vi "Configure Experiment.vi"(8 "Error In":errorcluster, 9 "KH":T4 {"KH #" items=["A 1", "A 2", "A 3", "A 4", "A 5", "A 6", "A 7", "A 8"]}, 10 "Lockin":T6 {"Label" items=["", "I+", "I-", "V1+", "V1-", "V2+", "V2-", "V3+", "V3-", "V4+", "V4-", "dV1", "dV2", "dV3", "Vsg", "Vbg", "Vtg"]}) -> (0 "Error Out":errorcluster)   [LabVIEW 2019, in "Control Experiment.lvclass"]
doc: "Use this VI to help configure your experiment.\n1. Configure the Electrode control to show which electrode is connected to which lockin channel;\n2. Choose a Label for each electrode to configure Krohn Hite amplifier automatically\n3. Easily set all Krohn Hite channels to be \"all ground\" or \"all differential\" mode\n4. Fill out information about you and your device in the lower left corner\n5. When you are finished, or when you want to update the amplifiers, click the \"CREATE OUTPUT\" button located in upper right. Clicking this button will set the amplifiers, and write information to a functional global variable that you can easily read from elsewhere in your program"
uses:
  Control Experiment.lvclass
  Typedefs/KH Mode-enum.ctl
  Typedefs/Control Experiment JSON--cluster.ctl
  <userlib>/LevyLab/Configuration/Configuration.lvclass
  Typedefs/UI Controls --cluster.ctl
  Typedefs/Instrument Types--enum.ctl
  Typedefs/Instruments--cluster.ctl
  <userlib>/LevyLab/Krohn Hite 7008/KH7008/typedefs/shunt--enum.ctl
  <userlib>/LevyLab/Krohn Hite 7008/KH7008/KH7008.lvlib
  <userlib>/LevyLab/Krohn Hite 7008/KH7008/typedefs/gain--enum.ctl
  <userlib>/LevyLab/Krohn Hite 7008/KH7008/typedefs/Input--Enum.ctl
  <userlib>/LevyLab/Krohn Hite 7008/KH7008/typedefs/channel--numeric.ctl
  <userlib>/LevyLab/Krohn Hite 7008/KH7008/typedefs/couple--Enum.ctl
  <userlib>/LevyLab/Krohn Hite 7008/KH7008/typedefs/Filter--Enum.ctl
  <userlib>/LevyLab/Krohn Hite 7008/KH7008/typedefs/channelProperties--Cluster.ctl
  <userlib>/LevyLab/Krohn Hite 7008/KH7008/typedefs/allChannelProperties--Array.ctl
  <userlib>/LevyLab/Krohn Hite 7008/Inst.Krohn-Hite-7008/Inst.Krohn-Hite-7008.lvclass
  Transport Server/Inst.Transport/Inst.Transport.lvclass
  Transport/Transport.lvclass
  <vilib>/JKI/JKI SMO/SMO/SMO.lvclass
  <userlib>/LevyLab/Instrument Framework/Instrument/Instrument.lvclass
  <userlib>/LevyLab/Instrument Framework/Instrument Types/Lockin/Instrument.LockinAPI.lvclass
  <userlib>/LevyLab/Instrument Framework/Instrument Types/VSource/Instrument.VSource.lvclass
  <userlib>/LevyLab/Instrument Framework/Instrument Types/VNA/Instrument.VNA.lvclass
  <userlib>/LevyLab/Instrument Framework/Instrument Types/Strain/Instrument.Strain.lvclass
  <userlib>/LevyLab/Instrument Framework/Instrument Types/Delay Line/Instrument.DelayLine.lvclass
  <userlib>/LevyLab/Instrument Framework/Instrument Types/CBridge/Instrument.CBridge.lvclass
  <userlib>/LevyLab/Instrument Framework/Instrument Types/Cryostat/Instrument.Cryostat.lvclass
  <userlib>/LevyLab/Instrument Framework/Instrument Types/Amplifier/Instrument.Amplifier.lvclass
  Typedefs/Instrument Classes--cluster.ctl
  C:/Program Files (x86)/National Instruments/LabVIEW 2019/vi.lib/JKI/JKI SMO/SMO/SMO.lvclass
  C:/Program Files (x86)/National Instruments/LabVIEW 2019/user.lib/LevyLab/Instrument Framework/Instrument/Instrument.lvclass
  C:/Program Files (x86)/National Instruments/LabVIEW 2019/user.lib/LevyLab/Instrument Framework/Instrument Types/Amplifier/Instrument.Amplifier.lvclass
  <vilib>/JKI/JKI SMO/URI Parsing/URI.lvlib
  b06a41f5-2f73-4e7a-a8dc-a6b31f20112d.vi
panel:
  in  "I'm Finished Taking Data!":bool
  out "State":string
  in  "Create Output":bool
  in  "String":string
  out "Values have changed":bool=TRUE
  in  "OK":bool
  out "Control Experiment":refnum<class "Control Experiment.lvclass">
  in  "C.E.":refnum<class "Control Experiment.lvclass">
  in  "Tab Control":enum32{"Input", "Output", "Configuration"}(tab)
  out "KH S/N":string
  out "MCL S/N":string
  in  "Transport Server":bool
  in  "Open KH7008":bool
  in  "Open Lockin":bool
  out "Lockin?":bool
  out "KH?":bool
  out "Transport?":bool
  in  "KH Chassis":i32 caption="AI Channels"
  in  "Type":u16(ring) items=["AFM", "EBL", "Cryo"]
  in  "Instrument Configuration":bool
  out "Configured Instruments":string
  in  "DC Coupled":bool=TRUE
  in  "BW Filter":bool=TRUE
  in  "AO Channels":u32=8
  in  "Gain":dbl[](array[numeric])=[1.0, 1.0, 1.0, 1.0, 1.0, 1.0, 1.0, 1.0, 1.0, 1.0, 1.0, 1.0, 1.0, 1.0, 1.0, 1.0]
  in  "AI Channels":u32=8
  in  "KH Configuration":T7(radio)
  in  "Default Resistor":T3=enum."5k"
  in  "Description":string
  in  "Sample (SAXXXX)":string
  in  "Device":string
  in  "Station":u16(ring) items=["CF900", "MNK", "PPMS (sim)", "Montana", "PPMS1", "PPMS2", "PPMS3", "OptiCool"]
  in  "User":u16(ring) items=["Jeremy", "Patrick", "Guanglei", "Juliana", "Ranjani", "Ahmed", "Yuhao", "Pubudu", "Sayanwita", "Aswini", "Aria", "Miles", "Bohao", "Sakshi"]
  in  "non KH":T8 {"Labels 2" items=["", "I+", "I-", "V1+", "V1-", "V2+", "V2-", "V3+", "V3-", "V4+", "V4-", "dV1", "dV2", "dV3", "Vsg", "Vbg", "Vtg"]}
  out "Device Folder":path=path "D:/Data/MNK/SA40178.20210125" caption="(\\base path\\project\\device\\ )"
  in  "Path":path=path "C:/temp" caption="Path (Typ. C:\\Users\\voodoo\\Nextcloud2\\Shared\\Instrument\\)"
  out "Comments":string
  out "JSON String":string
  in  "Label Strings":string
  # "Lockin"
  # "Krohn-Hite"
  # "Other"
  # "Channel and Chassis Configuration"
  # "Device and Project Description"
  # "Instrument Configuration"
  # "Apps"
  # "Path Configuration"
  # "Instructions: This application is used to configure your experiment\n\n1. Configure the Electrode control to show which electrode is connected to which lockin\n2. Choose a Label* for each electrode to configure Krohn Hite amplifier automatically\n3. Easily set all Krohn Hite channels to be \"all ground\" or \"all differential\" mode\n4. Fill out information about you and your device in the lower left corner\n5. When you are finished, or when you want to update the amplifiers, click the \"CONFIRM\" button located in upper right. Clicking this button will set the amplifiers and write information to a file that you can easily read from elsewhere in your program\n\n*If you want to have new labels for the \"Labels\" field you can type them below. Acceptable keywords are I, Vsg, Vbg, Vtg, dV, V, along with numeric indicies and +/-. Examples: V1+, V1-, dV1"
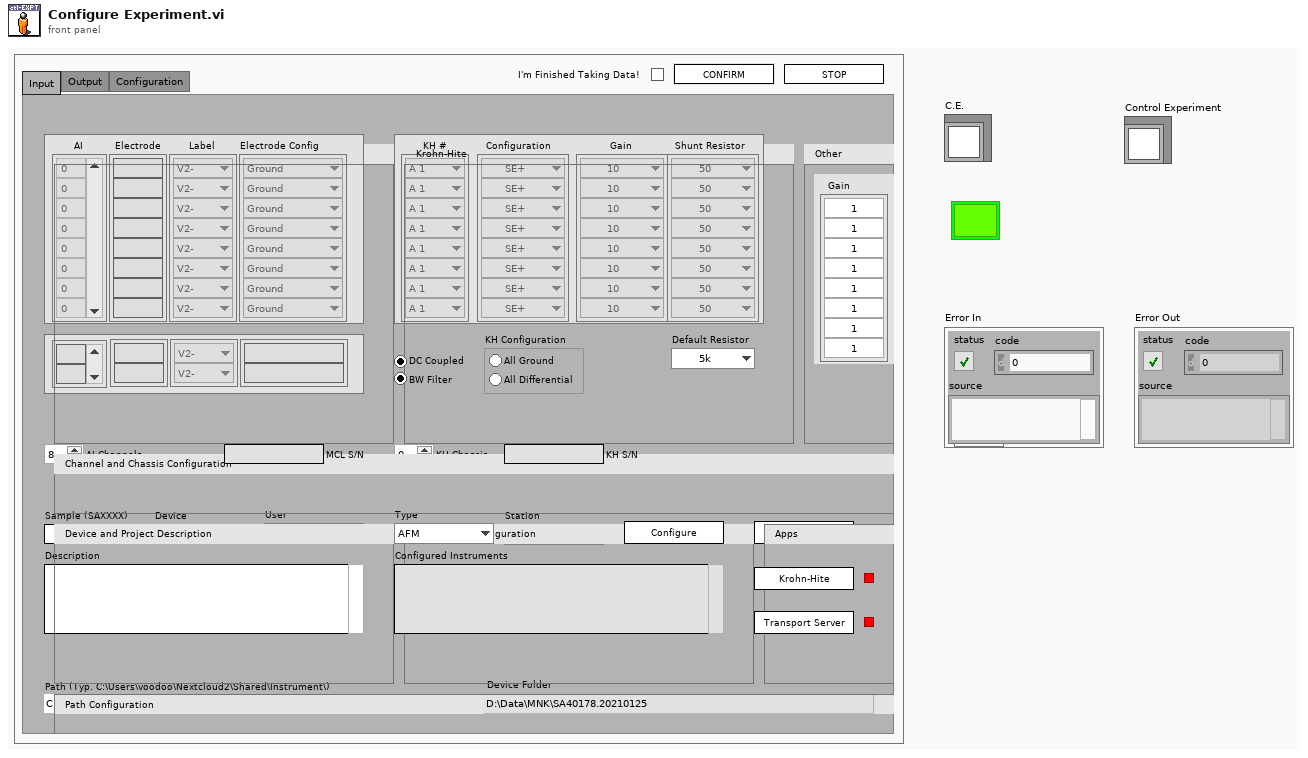
[diagram p1: front panel]
types:
  T1 = typedef "KH7008.lvlib/Input--Enum.ctl" = enum16{"OFF", "SE+", "SE-", "DIFF"}
  T2 = typedef "KH7008.lvlib/gain--enum.ctl" = enum16{"1", "10", "100", "1000"}
  T3 = typedef "KH7008.lvlib/shunt--enum.ctl" = enum16{"Open", "50", "500", "5k", "50k", "10M"}
  T4 = cluster{"KH #":u16[], "KH Configuration":T1[], "KH Gain":T2[], "KH Shunt Resistor":T3[]}
  T5 = typedef "Control Experiment.lvclass/KH Mode-enum.ctl" = enum16{"Ground", "Current", "Voltage (SE)", "Voltage (Diff)", "Gate"}
  T6 = cluster{"AI":u32[], "Electrode":string[], "Label":u16[], "Electrode Config":T5[]}
  T7 = enum32{"No Selection", "All Ground", "All Differential"}
  T8 = cluster{"Scroll Bar":string[], "Electrodes 2":string[], "Labels 2":u16[], "unused":string[]}
  T9 = enum32{"invalid app kind", "Development System", "Run Time System", "Student Edition", "Embedded LabVIEW", "Evaluation", "Custom"}
  T10 = enum32{"Bad", "Idle", "Run top level", "Running"}
  T11 = typedef "Control Experiment.lvclass/Instrument Classes--cluster.ctl" = cluster{"DAQ":refnum<class "Instrument.LockinAPI.lvclass">, "Amplifier":refnum<class "Instrument.Amplifier.lvclass">, "Temperature":refnum<class "Instrument.Cryostat.lvclass">, "Magnet":refnum<class "Instrument.Cryostat.lvclass">, "Rotator":refnum<class "Instrument.Cryostat.lvclass">, "Level":refnum<class "Instrument.Cryostat.lvclass">, "Capacitance":refnum<class "Instrument.CBridge.lvclass">, "Delay Line":refnum<class "Instrument.DelayLine.lvclass">, "Strain Cell":refnum<class "Instrument.Strain.lvclass">, "VNA":refnum<class "Instrument.VNA.lvclass">, "Source":refnum<class "Instrument.VSource.lvclass">}
  T12 = enum32{"Invalid", "Standard", "Closed", "Hidden", "Minimized", "Maximized"}
  T13 = typedef "KH7008.lvlib/channelProperties--Cluster.ctl" = cluster{"channel":T14, "gain":T2, "input":T1, "shunt":T3, "couple":T15, "filter":T16}
  T14 = typedef "KH7008.lvlib/channel--numeric.ctl" = u16
  T15 = typedef "KH7008.lvlib/couple--Enum.ctl" = enum16{"AC", "DC"}
  T16 = typedef "KH7008.lvlib/Filter--Enum.ctl" = enum16{"OFF", "ON"}
  T17 = typedef "Control Experiment.lvclass/Experiment Description--cluster.ctl" = cluster{"User":string, "Device":string, "Device Path":path, "Device Description":string, "Experiment Path":path, "Experiment Description":string, "Instrument":string, "Instruments":T18[], "Sweep":cluster{"key":string, "value":variant}[]}
  T18 = typedef "Control Experiment.lvclass/Instruments--cluster.ctl" = cluster{"class path":path, "Address":string, "Type":T19}
  T19 = typedef "Control Experiment.lvclass/Instrument Types--enum.ctl" = enum16{"DAQ", "Amplifier", "Temperature", "Magnet", "Rotator", "Level", "Capacitance", "Delay Line", "Strain Cell", "VNA", "Source"}
  T20 = typedef "Control Experiment.lvclass/Wiring Description--cluster.ctl" = cluster{"Lockin Ch":i32[], "KH":cluster{"Electrodes":string[], "Labels":string[]}, "not KH":cluster{"Electrodes":string[], "Labels":string[]}}
  T21 = typedef "KH7008.lvlib/allChannelProperties--Array.ctl" = T13[]
  T22 = typedef "Control Experiment.lvclass/UI Controls --cluster.ctl" = cluster{"Sample":string, "Device":string, "Username":string, "Description":string, "Default Path":path, "Instrument":string, "Station Type":string, "KH All Buttons":enum32{"No Selection", "All Ground", "All Differential"}, "Lockin":cluster{"AI":u32[], "Electrode":string[], "Label":u16[], "Electrode Config":T5[], "AI Channels":u32}, "KH":cluster{"KH #":enum16{"A 1", "A 2", "A 3", "A 4", "A 5", "A 6", "A 7", "A 8", "B 1", "B 2", "B 3", "B 4", "B 5", "B 6", "B 7", "B 8", "none"}[], "KH Configuration":T1[], "KH Gain":T2[], "KH Shunt Resistor":T3[], "Filter":bool, "DC Coupled":bool, "KH Chassis":i32}, "non KH":cluster{"Scroll Bar":string[], "Electrodes 2":string[], "Labels 2":u16[], "unused":string[]}, "Instrument Types":T18[]}
  T23 = cluster{"Core":cluster{"Current VI Reference":refnum<vi>, "Close Panel on Exit?":bool}, "C.E.":refnum<class "Control Experiment.lvclass">, "Experiment":T17, "Wiring Configuration":T20, "Channel Settings":cluster{"Channel Setting":T21}[], "KH Configuration":enum32{"No Selection", "All Ground", "All Differential"}, "Lockin":cluster{"AI":u32[], "Electrode":string[], "Label":u16[], "Electrode Config":T5[]}, "KH":cluster{"KH #":u16[], "KH Configuration":T1[], "KH Gain":T2[], "KH Shunt Resistor":T3[]}, "non KH":cluster{"Scroll Bar":string[], "Electrodes 2":string[], "Labels 2":u16[], "unused":string[]}, "UI":T22, "Config":refnum<class "Configuration.lvclass">, "Transport":refnum<class "Transport.lvclass">, "Transport-Server":refnum<class "Inst.Transport.lvclass">, "top level?":bool}
  T24 = typedef "SMO.lvclass/SMOState --Enum.ctl" = enum16{"unknown", "Created", "Started", "Stopped"}
  T25 = typedef "Inst.Transport.lvclass/UI State--enum.ctl" = enum16{"unknown", "Opened", "Closed"}
  T26 = cluster{"Current VI Reference":refnum<vi>, "Close Panel on Exit?":bool}
  T27 = typedef "SMO.lvclass/Public Events.ctl" = cluster{"Error":refnum<user-event>, "State":refnum<user-event>, "Reserve State":refnum<user-event>}
  T28 = typedef "Inst.Transport.lvclass/PublicEvents--Cluster.ctl" = cluster{"UI State":refnum<user-event>}
  T29 = cluster{"AI":u32[], "Electrode":string[], "Label":u16[], "Electrode Config":T5[], "AI Channels":u32}
  T30 = cluster{"KH #":enum16{"A 1", "A 2", "A 3", "A 4", "A 5", "A 6", "A 7", "A 8", "B 1", "B 2", "B 3", "B 4", "B 5", "B 6", "B 7", "B 8", "none"}[], "KH Configuration":T1[], "KH Gain":T2[], "KH Shunt Resistor":T3[], "Filter":bool, "DC Coupled":bool, "KH Chassis":i32}
  T31 = enum16{"A 1", "A 2", "A 3", "A 4", "A 5", "A 6", "A 7", "A 8", "B 1", "B 2", "B 3", "B 4", "B 5", "B 6", "B 7", "B 8", "none"}[]
  T32 = typedef "Control Experiment.lvclass/Control Experiment JSON--cluster.ctl" = cluster{"Device":cluster{"Device":string, "User":string, "Time":string, "Computer Name":string}, "Wiring":cluster{"Lockin Ch":u32[], "KH Electrodes":string[], "KH Labels":string[], "Other Electrodes":string[], "Other Labels":string[]}}
  T33 = typedef "Instrument.lvlib/Instrument.lvclass/Instrument.IDN--cluster.ctl" = cluster{"vendor":string, "model":string, "serial":string, "firmware":string}
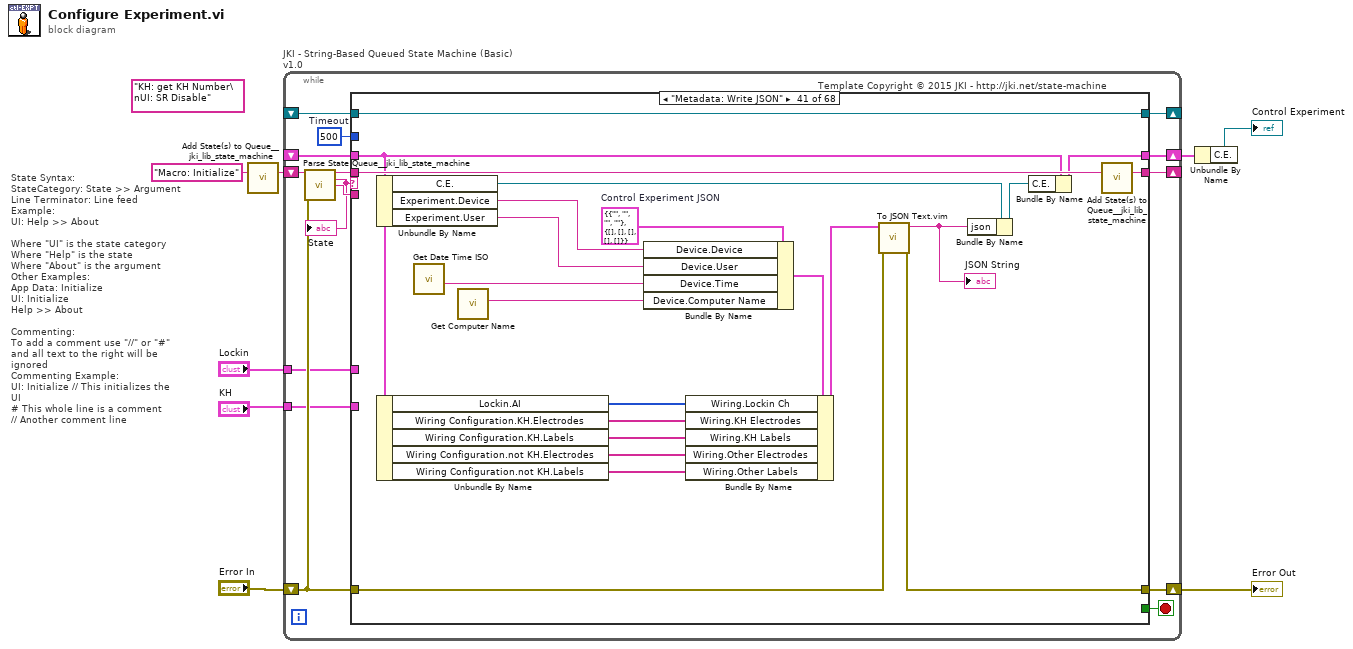
[diagram p0: block diagram]
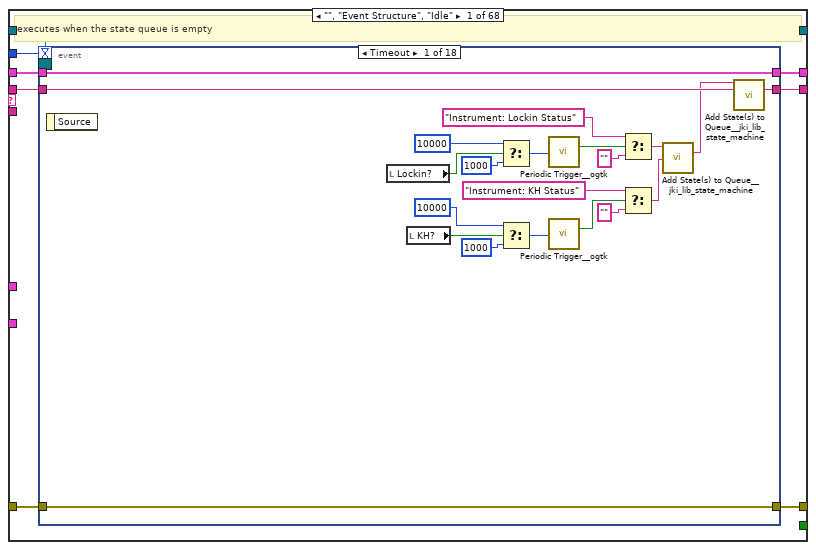
[diagram p2: hidden frame]
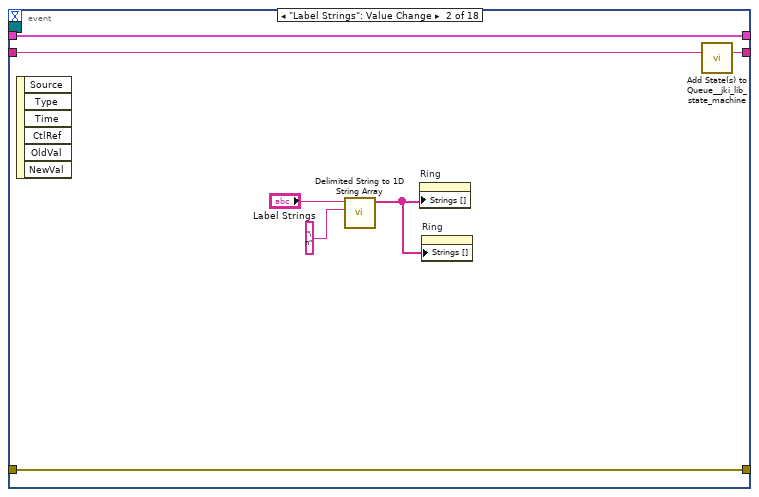
[diagram p3: hidden frame]
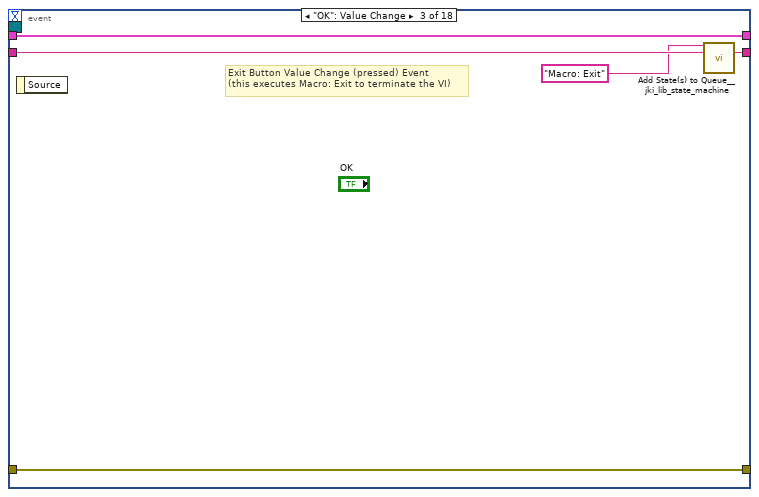
[diagram p4: hidden frame]
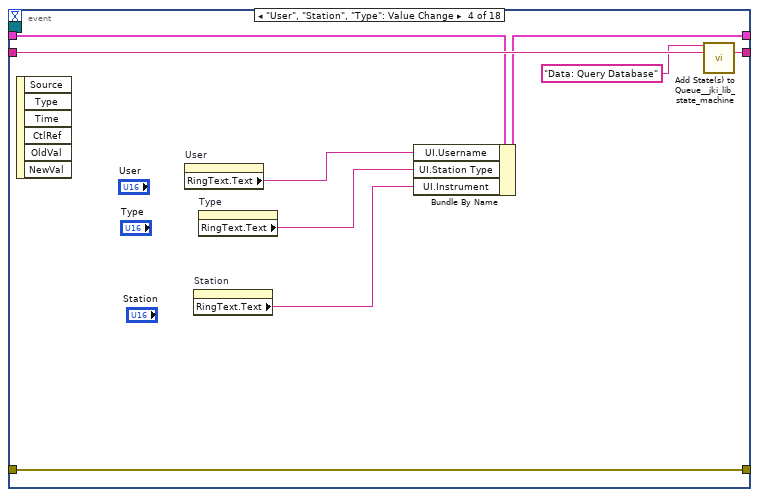
[diagram p5: hidden frame]
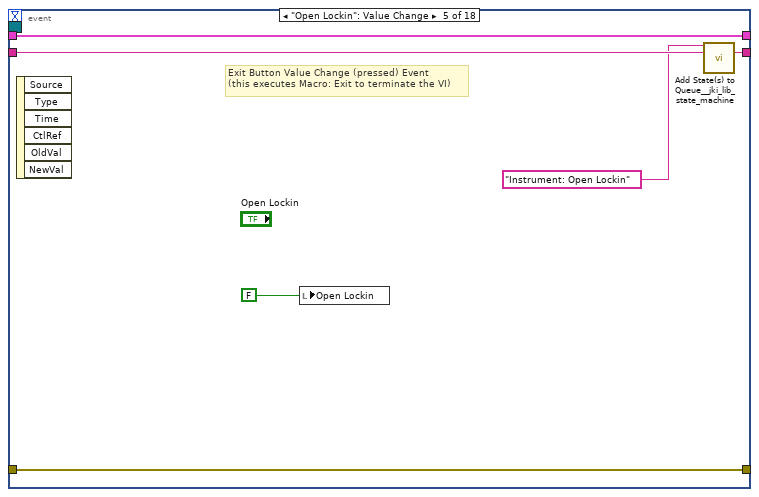
[diagram p6: hidden frame]
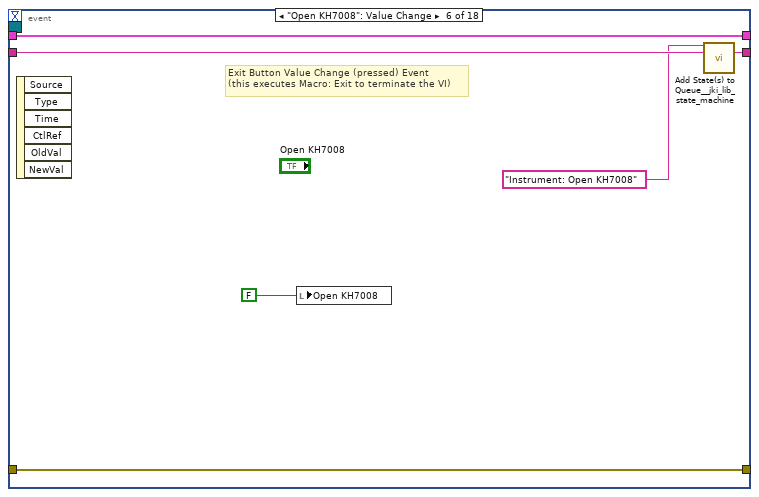
[diagram p7: hidden frame]
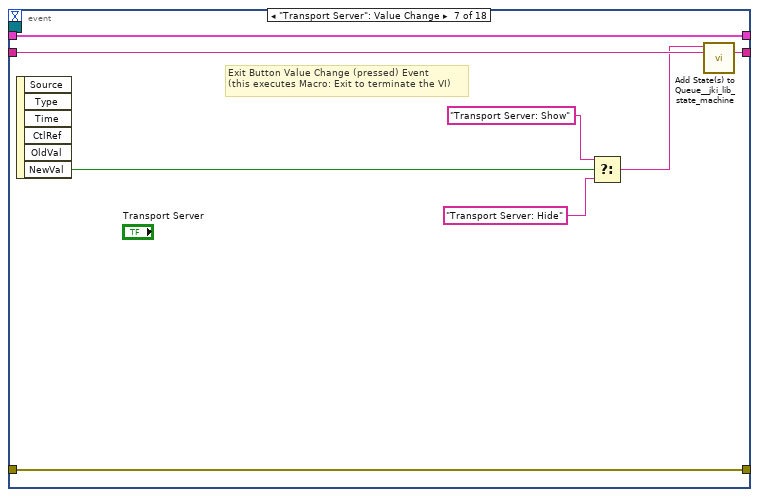
[diagram p8: hidden frame]
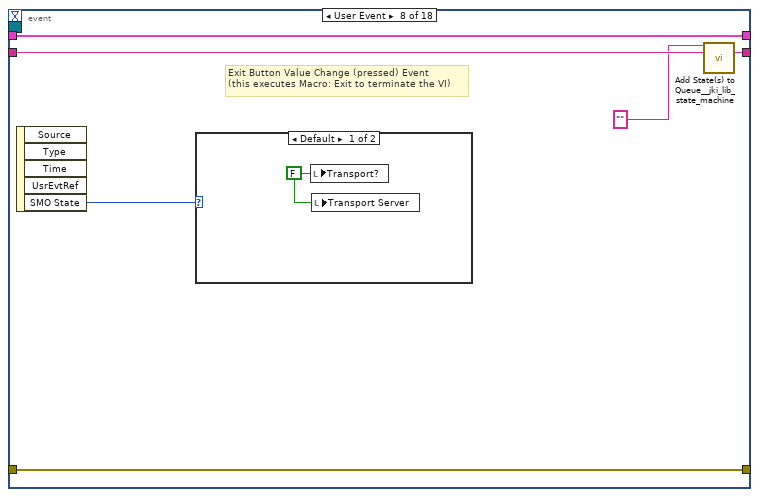
[diagram p9: hidden frame]
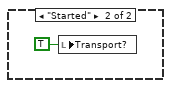
[diagram p10: hidden frame]
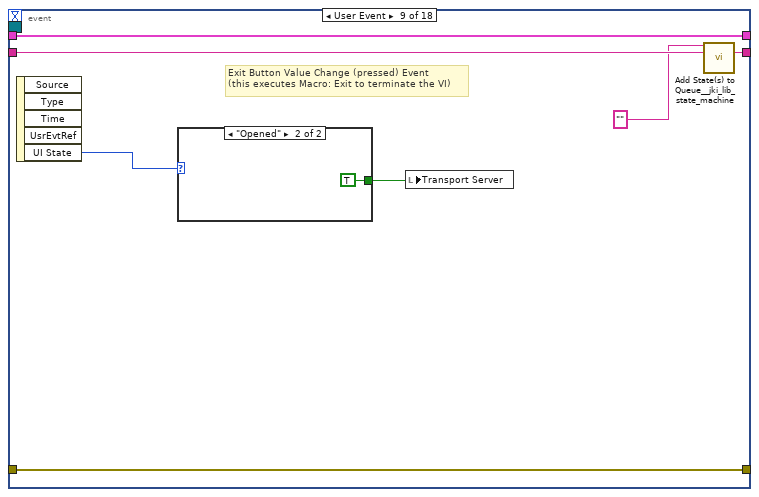
[diagram p11: hidden frame]
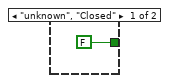
[diagram p12: hidden frame]
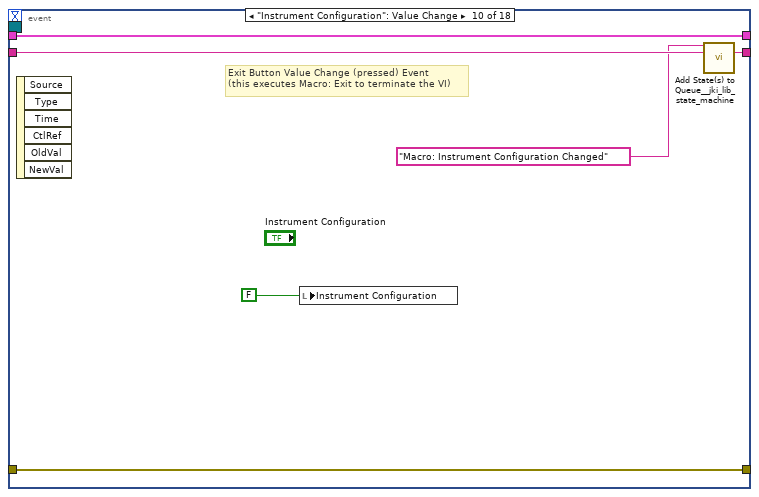
[diagram p13: hidden frame]
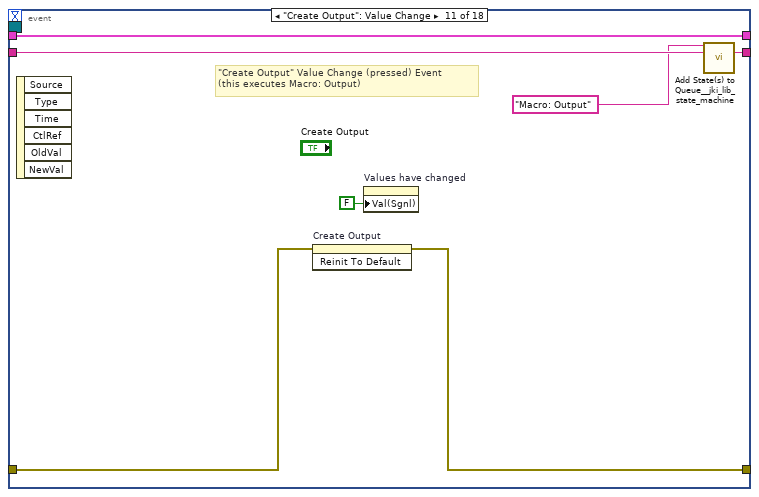
[diagram p14: hidden frame]
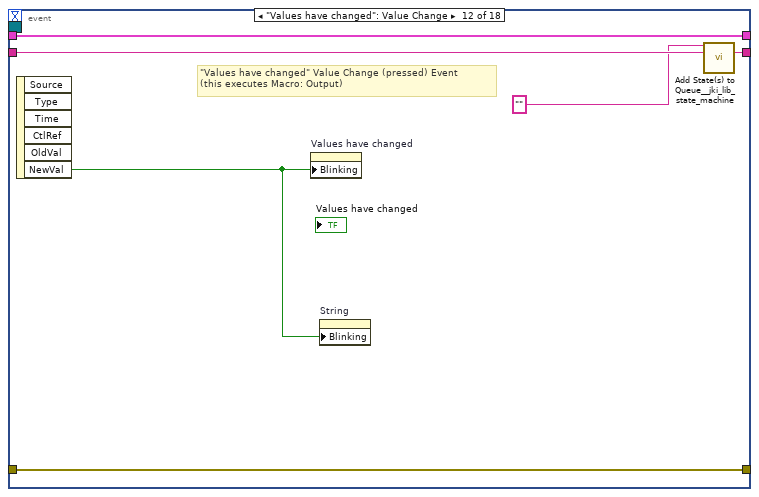
[diagram p15: hidden frame]
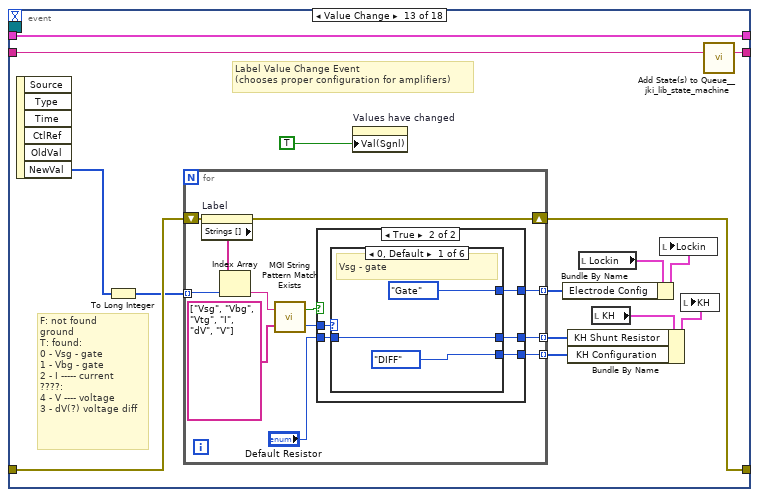
[diagram p16: hidden frame]
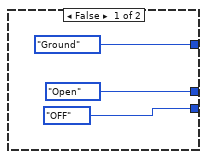
[diagram p17: hidden frame]
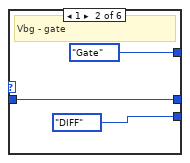
[diagram p18: hidden frame]
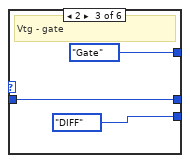
[diagram p19: hidden frame]
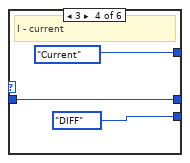
[diagram p20: hidden frame]
diagram:
  (unwired) "KH: get KH Number\nUI: SR Disable" ("State(s) in Front (\"\")")
  # "State Syntax:\nStateCategory: State >> Argument\nLine Terminator: Line feed\nExample:\nUI: Help >> About\n\nWhere \"UI\" is the state category\nWhere \"Help\" is the state\nWhere \"About\" is the argument\nOther Examples:\nApp Data: Initialize\nUI: Initialize\nHelp >> About\n\nCommenting:\nTo add a comment use \"//\" or \"#\" and all text to the right will be ignored\nCommenting Example:\nUI: Initialize // This initializes the UI\n# This whole line is a comment\n// Another comment line"
  n1 = call <vilib>:"Add State(s) to Queue__jki_lib_state_machine.vi"("State(s) in (\"\")"="Macro: Initialize") -> ("States Out"=w8:string)  [unwired: 14 in]
  n2 = while "JKI - String-Based Queued State Machine (Basic) v1.0" {
    shift-right: [w17] -> w6
    shift-left: _ -> [w16]
    shift-right: [w20] -> w2
    shift-left: "Error In" -> [w14]
    shift-right: [w19] -> _
    shift-left: w8 -> [w21]
    tunnel: "Lockin" -> [w13]
    tunnel: "KH" -> [w12]
    shift-right: [w10] -> _
    shift-left: _ -> [w9]
    stop <- w18 stop-if-true
    w15 = 500  # Timeout
    # "Template Copyright © 2015 JKI - http://jki.net/state-machine"
    n3 = call <vilib>:"Parse State Queue__jki_lib_state_machine.vi"("State Queue"=w21, "Error In (no error)"=w14) -> ("Remaining States"=w23:string, "Current State"=w11:string, "Arguments"=w22:string)  [unwired: 11 in]
    "State" <- w11
    n4 = case shown="\"Metadata: Write JSON\"" w11 {
      selector: w11 -> [_ _ w234 _ _ _ _ _ _ _ _ _ _ _ _ _ _ _ _ _ _ _ _ _ _ _ _ _ _ _ _ _ _ _ _ _ _ _ _ _ _ _ _ _ _ _ _ _ _ _ _ _ _ _ _ _ _ _ _ _ _ _ _ _ _ _ _ _]
      tunnel: w23 -> [w31 w232 w238 w257 w264 w270 w275 w294 w306 w322 w354 w361 w391 w396 w409 w415 w420 w442 w473 w493 w529 w541 w568 w584 w599 w620 w626 w638 w646 w653 w659 w665 w670 w683 w702 w727 w787 w840 w850 w862 w884 w892 w901 w906 w921 w955 w1047 w1092 w1113 w1129 w1138 w1143 w1162 w1198 w1226 w1258 w1264 w1269 w1280 w1289 w1298 w1307 w1315 w1323 w1328 w1344 w1349 w1357]
      tunnel: w22 -> [_ _ _ _ _ _ _ _ _ _ _ _ _ _ _ _ _ _ _ _ w524 w535 _ _ _ _ _ _ _ _ _ _ _ _ _ _ _ _ _ _ _ _ _ _ _ _ _ _ _ _ _ _ _ _ _ _ _ _ _ _ _ _ _ _ _ _ _ w1352]
      tunnel: w16 -> [w29 w229 w236 w248 w261 w268 w272 _ w301 w308 w334 w358 w383 w393 w407 w413 w417 w435 w462 w491 w527 w537 w565 w581 w597 w617 w623 w635 w644 w650 w656 w662 w667 w679 w698 w725 w785 w838 w846 w860 w870 w890 w894 w903 w919 w947 w1042 w1087 w1109 w1126 w1136 w1140 w1153 w1193 w1221 w1256 w1262 w1266 w1277 w1282 w1294 w1301 w1312 w1320 w1325 w1342 w1346 w1354]
      tunnel: [w28 w230 w240 w254 errorcluster {"status"=FALSE, "code"=0, "source"=""} ("error out") w267 w273 w291 w304 w319 w344 w359 w389 w394 w403 w410 w418 w423 w471 w486 w525 w538 w566 w582 w589 w618 w624 w636 w642 w651 w657 w663 w668 w681 w700 w718 w780 w833 w843 w853 w866 w887 w898 w904 w911 w946 w1044 w1085 w1110 w1127 w1131 w1141 w1160 w1196 w1224 w1254 w1260 w1267 w1271 w1285 w1290 w1304 w1311 w1319 w1326 w1334 w1347 w1355] -> w20
      tunnel: w14 -> [w27 w230 w239 w254 w260 w267 w273 w291 w304 w320 w345 w356 w389 w394 w402 w411 w418 w440 w471 w486 w526 w539 w566 w582 w590 w618 w624 w636 w642 w651 w657 w663 w668 w681 w700 w715 w777 w834 w843 w854 w872 w886 w897 w904 w909 w946 w1037 w1084 w1106 w1127 w1133 w1141 w1160 w1196 w1224 w1255 w1261 w1267 w1273 w1284 w1291 w1303 w1310 w1318 w1326 w1335 w1347 w1355]
      tunnel: [w30 w231 w237 w256 w263 w269 w274 w293 w305 w321 w353 w360 w390 w395 w408 w414 w419 w441 w472 w492 w528 w540 w567 w583 w598 w619 w625 w637 w645 w652 w658 w664 w669 w682 w701 w726 w786 w839 w849 w861 w883 w891 w900 w905 w920 w954 w1046 w1091 w1112 w1128 w1137 w1142 w1161 w1197 w1225 w1257 w1263 w1268 w1279 w1288 w1297 w1306 w1314 w1322 w1327 w1343 w1348 w1356] -> w19
      tunnel: [_ _ _ _ _ TRUE _ _ _ _ _ _ _ _ _ _ _ _ _ _ _ _ _ _ _ _ _ _ _ _ _ _ _ _ _ _ _ _ _ _ _ _ _ _ _ _ _ _ _ _ _ _ _ _ _ _ _ _ _ _ _ _ _ _ _ _ _ _] -> w18
      tunnel: [w26 w229 w236 w255 w261 w268 w272 w292 w300 w307 w335 w358 w384 w393 w407 w413 w417 w435 w462 w491 w527 w537 w565 w581 w597 w617 w623 w635 w644 w650 w656 w662 w667 w680 w699 w711 w771 w837 w845 w859 w871 w890 w895 w903 w918 w953 w1045 w1087 w1111 w1126 w1135 w1140 w1154 w1194 w1222 w1256 w1262 w1266 w1278 w1283 w1295 w1302 w1313 w1321 w1325 w1342 w1346 w1354] -> w17
      tunnel: w15 -> [w25 _ _ _ _ _ _ _ _ _ _ _ _ _ _ _ _ _ _ _ _ _ _ _ _ _ _ _ _ _ _ _ _ _ _ _ _ _ _ _ _ _ _ _ _ _ _ _ _ _ _ _ _ _ _ _ _ _ _ _ _ _ _ _ _ _ _ _]
      tunnel: w13 -> [_ _ _ _ _ _ _ w280 _ _ _ _ _ _ _ _ _ _ _ _ _ _ _ _ _ _ _ _ _ _ _ _ _ _ _ _ _ _ _ _ _ _ _ _ _ _ _ _ _ _ _ _ _ _ _ _ _ _ _ _ _ _ _ _ _ _ _ _]
      tunnel: w12 -> [_ _ _ _ _ _ _ w279 _ _ _ _ _ _ _ _ _ _ _ _ _ _ _ _ _ _ _ _ _ _ _ _ _ _ _ _ _ _ _ _ _ _ _ _ _ _ _ _ _ _ _ _ _ _ _ _ _ _ _ _ _ _ _ _ _ _ _ _]
      tunnel: [w24 w228 w233 w245 w258 w265 w271 w276 w295 w318 w323 w355 w362 w392 w401 w412 w416 w432 w444 w485 w523 w534 w564 w569 w596 w616 w621 w627 w639 w648 w654 w660 w666 w671 w686 w709 w770 w830 w841 w851 w863 w885 w893 w902 w907 w935 w1026 w1077 w1100 w1125 w1130 w1139 w1159 w1195 w1223 w1253 w1259 w1265 w1276 w1281 w1293 w1299 w1309 w1317 w1324 w1333 w1345 w1353] -> w10
      tunnel: w9 -> [w24 w228 w233 w245 w258 w265 w271 w276 w295 w318 w323 w355 w362 w392 _ w412 w416 w432 w444 w485 w523 w534 w564 w569 w596 w616 w621 w627 w639 w648 w654 w660 w666 w671 w686 w709 w770 w830 w841 w851 w863 w885 w893 w902 w907 w935 w1026 w1077 w1100 w1125 w1130 w1139 w1159 w1195 w1223 w1253 w1259 w1265 w1276 w1281 w1293 w1299 w1309 w1317 w1324 w1333 w1345 w1353]
      frame "", "Event Structure", "Idle" {
        # "executes when the state queue is empty"
        n5 = event shown="[0] Timeout" {
          selector: w24 -> [_ _ _ _ _ _ _ _ _ _ _ _ _ _ _ _ _ _]
          dyn-events: _ -> [_ _ _ _ _ _ _ _ _ _ _ _ _ _ _ _ _ _]
          timeout: w25 -> [_ _ _ _ _ _ _ _ _ _ _ _ _ _ _ _ _ _]
          tunnel: w31 -> [w52 w57 w64 w73 w79 w85 w93 w99 w108 w116 w123 w129 w144 w184 w189 w207 w213 w227]
          tunnel: [w51 w59 w63 w72 w78 w84 w92 w98 w107 w115 w122 w128 w143 w184 w188 w206 w215 w226] -> w30
          tunnel: w29 -> [w49 w58 w61 w68 w76 w82 w90 w96 w105 w113 w121 w127 w142 w185 w190 w205 w216 w224]
          tunnel: [w50 w56 w62 w71 w77 w83 w91 w97 w106 w114 w118 w125 w133 w186 w191 w208 w212 w225] -> w28
          tunnel: w27 -> [w50 w56 w62 w71 w77 w83 w91 w97 w106 w114 w119 w125 w140 w186 w191 w208 w212 w225]
          tunnel: [w49 w58 w61 w69 w76 w82 w90 w96 w105 w113 w121 w127 w142 w185 w190 w205 w216 w224] -> w26
          event Timeout {
            n6 = event-data() -> ()  [unwired: 1 in, 1 out]
            n7 = local read "Lockin?"() -> (w36:bool)
            n8 = local read "KH?"() -> (w37:bool)
            n9 = Select(t=u32 10000 ("time (ms)"), s=w36, f=u32 1000) -> (s? t:f=w39:u32)
            n10 = Select(t=u32 10000 ("time (ms)"), s=w37, f=u32 1000) -> (s? t:f=w38:u32)
            n11 = call <userlib>:"Periodic Trigger__ogtk.vi"("time (ms)"=w39) -> ("Triggered"=w33:bool)  [unwired: 12 in, 2 out]
            n12 = call <userlib>:"Periodic Trigger__ogtk.vi"("time (ms)"=w38) -> ("Triggered"=w32:bool)  [unwired: 12 in, 2 out]
            n13 = Select(t="Instrument: Lockin Status", s=w33, f="") -> (s? t:f=w43:string)
            n14 = Select(t="Instrument: KH Status", s=w32, f="") -> (s? t:f=w46:string)
            n15 = call <vilib>:"Add State(s) to Queue__jki_lib_state_machine.vi"("State(s) in Front (\"\")"=w43, "State(s) at Back (\"\")"=w46) -> ("States Out"=w42:string)  [unwired: 13 in]
            n16 = call <vilib>:"Add State(s) to Queue__jki_lib_state_machine.vi"("State(s) in Front (\"\")"=w42, "State(s) in (\"\")"=w52) -> ("States Out"=w51:string)  [unwired: 13 in]
          }
          event "Label Strings": Value Change {
            n17 = event-data() -> ()  [unwired: 1 in, 6 out]
            n18 = call <vilib>:"Delimited String to 1D String Array.vi"("delimiter"="\n", "delimited string"="Label Strings") -> ("string array"=w54:string[])  [unwired: 9 in]
            n19 = property on="Ring" class="Ring (strict)"("Strings []"=w54) -> ()  [unwired: 2 in, 2 out]
            n20 = property on="Ring" class="Ring (strict)"("Strings []"=w54) -> ()  [unwired: 2 in, 2 out]
            n21 = call <vilib>:"Add State(s) to Queue__jki_lib_state_machine.vi"("State(s) in (\"\")"=w57) -> ("States Out"=w59:string)  [unwired: 14 in]
          }
          event "OK": Value Change {
            # "Exit Button Value Change (pressed) Event\n(this executes Macro: Exit to terminate the VI)"
            n22 = event-data() -> ()  [unwired: 1 in, 1 out]
            n23 = call <vilib>:"Add State(s) to Queue__jki_lib_state_machine.vi"("State(s) in Front (\"\")"="Macro: Exit", "State(s) in (\"\")"=w64) -> ("States Out"=w63:string)  [unwired: 13 in]
          }
          event "User", "Station", "Type": Value Change {
            n24 = event-data() -> ()  [unwired: 1 in, 6 out]
            n25 = property on="User" class="Ring (strict)"() -> ("RingText.Text"=w67:string)  [unwired: 2 in, 2 out]
            n26 = property on="Station" class="Ring (strict)"() -> ("RingText.Text"=w66:string)  [unwired: 2 in, 2 out]
            n27 = property on="Type" class="Ring (strict)"() -> ("RingText.Text"=w65:string)  [unwired: 2 in, 2 out]
            n28 = Bundle By Name(cluster=w68, "UI.Username"=w67, "UI.Station Type"=w65, "UI.Instrument"=w66) -> (w69:T23)
            n29 = call <vilib>:"Add State(s) to Queue__jki_lib_state_machine.vi"("State(s) in Front (\"\")"="Data: Query Database", "State(s) in (\"\")"=w73) -> ("States Out"=w72:string)  [unwired: 13 in]
          }
          event "Open Lockin": Value Change {
            # "Exit Button Value Change (pressed) Event\n(this executes Macro: Exit to terminate the VI)"
            n30 = event-data() -> ()  [unwired: 1 in, 6 out]
            n31 = local write "Open Lockin"(FALSE ("Open VI")) -> ()
            n32 = call <vilib>:"Add State(s) to Queue__jki_lib_state_machine.vi"("State(s) in Front (\"\")"="Instrument: Open Lockin", "State(s) in (\"\")"=w79) -> ("States Out"=w78:string)  [unwired: 13 in]
          }
          event "Open KH7008": Value Change {
            # "Exit Button Value Change (pressed) Event\n(this executes Macro: Exit to terminate the VI)"
            n33 = event-data() -> ()  [unwired: 1 in, 6 out]
            n34 = local write "Open KH7008"(FALSE ("Open VI")) -> ()
            n35 = call <vilib>:"Add State(s) to Queue__jki_lib_state_machine.vi"("State(s) in Front (\"\")"="Instrument: Open KH7008", "State(s) in (\"\")"=w85) -> ("States Out"=w84:string)  [unwired: 13 in]
          }
          event "Transport Server": Value Change {
            # "Exit Button Value Change (pressed) Event\n(this executes Macro: Exit to terminate the VI)"
            n36 = event-data() -> ("NewVal"=w86:bool)  [unwired: 1 in, 5 out]
            n37 = Select(t="Transport Server: Show", s=w86, f="Transport Server: Hide") -> (s? t:f=w87:string)
            n38 = call <vilib>:"Add State(s) to Queue__jki_lib_state_machine.vi"("State(s) in Front (\"\")"=w87, "State(s) in (\"\")"=w93) -> ("States Out"=w92:string)  [unwired: 13 in]
          }
          event User Event {
            # "Exit Button Value Change (pressed) Event\n(this executes Macro: Exit to terminate the VI)"
            n39 = event-data() -> ("SMO State"=w94:T24)  [unwired: 1 in, 4 out]
            n40 = case shown="Default" w94 {
              frame Default {
                w100 = FALSE ("Transport?")
                n41 = local write "Transport?"(w100) -> ()
                n42 = local write "Transport Server"(w100) -> ()
              }
              frame "Started" {
                n43 = local write "Transport?"(TRUE ("Transport?")) -> ()
              }
            }
            n44 = call <vilib>:"Add State(s) to Queue__jki_lib_state_machine.vi"("State(s) in Front (\"\")"="" ("State(s) in Front (\"\")"), "State(s) in (\"\")"=w99) -> ("States Out"=w98:string)  [unwired: 13 in]
          }
          event User Event {
            # "Exit Button Value Change (pressed) Event\n(this executes Macro: Exit to terminate the VI)"
            n45 = event-data() -> ("UI State"=w103:T25)  [unwired: 1 in, 4 out]
            n46 = case shown="\"Opened\"" w103 {
              tunnel: [FALSE ("Transport Server") TRUE ("Transport Server")] -> w102
              frame "unknown", "Closed" {
              }
              frame "Opened" {
              }
            }
            n47 = local write "Transport Server"(w102) -> ()
            n48 = call <vilib>:"Add State(s) to Queue__jki_lib_state_machine.vi"("State(s) in Front (\"\")"="" ("State(s) in Front (\"\")"), "State(s) in (\"\")"=w108) -> ("States Out"=w107:string)  [unwired: 13 in]
          }
          event "Instrument Configuration": Value Change {
            # "Exit Button Value Change (pressed) Event\n(this executes Macro: Exit to terminate the VI)"
            n49 = event-data() -> ()  [unwired: 1 in, 6 out]
            n50 = local write "Instrument Configuration"(FALSE ("Open VI")) -> ()
            n51 = call <vilib>:"Add State(s) to Queue__jki_lib_state_machine.vi"("State(s) in Front (\"\")"="Macro: Instrument Configuration Changed", "State(s) in (\"\")"=w116) -> ("States Out"=w115:string)  [unwired: 13 in]
          }
          event "Create Output": Value Change {
            # "\"Create Output\" Value Change (pressed) Event\n(this executes Macro: Output)"
            n52 = event-data() -> ()  [unwired: 1 in, 6 out]
            n53 = invoke on="Create Output" class="Bool" method="Reinit To Default"(error in=w119) -> (error out=w118:errorcluster)  [unwired: 2 in, 2 out]
            n54 = property on="Values have changed" class="Bool (strict)"("Val(Sgnl)"=FALSE ("Value (Signaling)")) -> ()  [unwired: 2 in, 2 out]
            n55 = call <vilib>:"Add State(s) to Queue__jki_lib_state_machine.vi"("State(s) in Front (\"\")"="Macro: Output", "State(s) in (\"\")"=w123) -> ("States Out"=w122:string)  [unwired: 13 in]
          }
          event "Values have changed": Value Change {
            # "\"Values have changed\" Value Change (pressed) Event\n(this executes Macro: Output)"
            n56 = event-data() -> ("NewVal"=w124:bool)  [unwired: 1 in, 5 out]
            n57 = property on="Values have changed" class="Bool (strict)"("Blinking"=w124) -> ()  [unwired: 2 in, 2 out]
            n58 = property on="String" class="Str"("Blinking"=w124) -> ()  [unwired: 2 in, 2 out]
            n59 = call <vilib>:"Add State(s) to Queue__jki_lib_state_machine.vi"("State(s) in Front (\"\")"="", "State(s) in (\"\")"=w129) -> ("States Out"=w128:string)  [unwired: 13 in]
          }
          event "Lockin.Label": Value Change {
            # "F: not found\nground\nT: found:\n0 - Vsg - gate\n1 - Vbg - gate\n2 - I ----- current\n????:\n4 - V ---- voltage\n3 - dV(?) voltage diff"
            # "Label Value Change Event\n(chooses proper configuration for amplifiers)"
            n60 = event-data() -> ("NewVal"=w141:u16[])  [unwired: 1 in, 5 out]
            n61 = To Long Integer(number=w141) -> (32bit integer=w130:i32[])
            n62 = for {
              tunnel: w130 -> [w153] mode=indexing
              tunnel: [w155] -> w137 mode=indexing
              tunnel: [w150] -> w134 mode=indexing
              tunnel: [w146] -> w135 mode=indexing
              shift-right: [w151] -> w133
              shift-left: w140 -> [w152]
              n63 = property on="Label" class="Ring (strict)"(error in=w152) -> (error out=w151:errorcluster, "Strings []"=w154:string[])  [unwired: 1 in, 1 out]
              n64 = Index Array(array=w154, index=w153) -> (element=w149:string)
              n65 = call <userlib>:"MGI String Pattern Match Exists.vi"("Patterns to Try"=string[] ["Vsg", "Vbg", "Vtg", "I", "dV", "V"], "String"=w149) -> ("Index of First Pattern Matched"=w156:i32, "Match Found"=w147:bool)
              n66 = case shown="True" w147 {
                tunnel: w156 -> [_ w164]
                tunnel: [KH_Mode-enum."Ground" ("Enum") w163] -> w155
                tunnel: [shunt--enum."Open" ("Shunt Resistor") w162] -> w150
                tunnel: [Input--Enum."OFF" ("Input Configuation") w161] -> w146
                tunnel: "Default Resistor" -> [_ w160]
                frame False {
                }
                frame True {
                  n67 = case shown="0, Default" w164 {
                    tunnel: [KH_Mode-enum."Gate" ("Enum") KH_Mode-enum."Gate" ("Enum") KH_Mode-enum."Gate" ("Enum") KH_Mode-enum."Current" ("Enum") KH_Mode-enum."Voltage (Diff)" ("Enum") KH_Mode-enum."Voltage (SE)" ("Enum")] -> w163
                    tunnel: [w165 w168 w171 w174 shunt--enum."Open" ("Shunt Resistor") shunt--enum."Open" ("Shunt Resistor")] -> w162
                    tunnel: [Input--Enum."DIFF" ("Input Configuation") Input--Enum."DIFF" ("Input Configuation") Input--Enum."DIFF" ("Input Configuation") Input--Enum."DIFF" ("Input Configuation") Input--Enum."DIFF" ("Input Configuation") Input--Enum."SE+" ("Input Configuation")] -> w161
                    tunnel: w160 -> [w165 w168 w171 w174 _ _]
                    frame 0, Default {
                      # "Vsg - gate"
                    }
                    frame 1 {
                      # "Vbg - gate"
                    }
                    frame 2 {
                      # "Vtg - gate"
                    }
                    frame 3 {
                      # "I - current"
                    }
                    frame 4 {
                      # "dV - V (Diff)"
                    }
                    frame 5 {
                      # "V - V (SE)"
                    }
                  }
                }
              }
            }
            n68 = property on="Values have changed" class="Bool (strict)"("Val(Sgnl)"=TRUE ("Values have changed")) -> ()  [unwired: 2 in, 2 out]
            n69 = local read "Lockin"() -> (w138:T6)
            n70 = Bundle By Name(cluster=w138, "Electrode Config"=w137) -> (w132:T6)
            n71 = local read "KH"() -> (w136:T4)
            n72 = Bundle By Name(cluster=w136, "KH Shunt Resistor"=w134, "KH Configuration"=w135) -> (w131:T4)
            n73 = local write "Lockin"(w132) -> ()
            n74 = local write "KH"(w131) -> ()
            n75 = call <vilib>:"Add State(s) to Queue__jki_lib_state_machine.vi"("State(s) in (\"\")"=w144) -> ("States Out"=w143:string)  [unwired: 14 in]
          }
          event "KH.KH Shunt Resistor", "KH.KH Gain", "non KH.Electrodes 2", "non KH.Labels 2", "Sample (SAXXXX)", "Description", "Lockin.Electrode": Value Change {
            n76 = event-data() -> ()  [unwired: 1 in, 6 out]
            n77 = property on="Values have changed" class="Bool (strict)"("Val(Sgnl)"=TRUE ("Values have changed")) -> ()  [unwired: 2 in, 2 out]
          }
          event "Lockin.AI", "non KH.Scroll Bar": Mouse Move; "Lockin.AI", "non KH.Scroll Bar": Mouse Wheel {
            n78 = event-data() -> ()  [unwired: 1 in, 5 out]
            n79 = call <vilib>:"Add State(s) to Queue__jki_lib_state_machine.vi"("State(s) in Front (\"\")"="UI: Link Scroll Bars" ("State(s) in Front (\"\")"), "State(s) in (\"\")"=w189) -> ("States Out"=w188:string)  [unwired: 13 in]
          }
          event "AI Channels": Value Change {
            n80 = event-data() -> ("NewVal"=w193:u32)  [unwired: 1 in, 5 out]
            n81 = To Long Integer(number=w193) -> (32bit integer=w192:i32)
            n82 = for {
              N: w192 -> [_]
              tunnel: [w211] -> w197 mode=indexing
              tunnel: [w210] -> w196 mode=indexing
              i -> [w210]
              n83 = Increment(x=w210) -> (x+1=w211:i32)
            }
            n84 = local read "Lockin"() -> (w204:T6)
            n85 = Initialize Array(1.0 ("element"), w192) -> (w200:dbl[])
            n86 = Bundle By Name(cluster=w204, "AI"=w197) -> (w203:T6)
            n87 = for {
              N: w192 -> [_]
              tunnel: [w209] -> w194 mode=indexing
              i -> [w209]
            }
            n88 = local read "KH"() -> (w199:T4)
            n89 = local write "Gain"(w200) -> ()
            n90 = control-ref of="KH #"() -> (w195:refnum<vi>)
            n91 = Bundle By Name(cluster=w199, "KH #"=w196) -> (w202:T4)
            n92 = local write "Lockin"(w203) -> ()
            n93 = local write "KH"(w202) -> ()
            n94 = property on="Property Node" class="Arr (strict)"(reference=w195, "Value"=w194) -> ()  [unwired: 1 in, 2 out]
            n95 = call <vilib>:"Add State(s) to Queue__jki_lib_state_machine.vi"("State(s) in Front (\"\")"="Metadata: Update AI\nMetadata: Update KH\nKH: set KH 0\nKH: set KH 1" ("State(s) in Front (\"\")"), "State(s) in (\"\")"=w207) -> ("States Out"=w206:string)  [unwired: 13 in]
          }
          event "KH Chassis": Value Change {
            n96 = event-data() -> ("NewVal"=w217:i32)  [unwired: 1 in, 5 out]
            n97 = local write "KH Chassis"(w217) -> ()
            n98 = call <vilib>:"Add State(s) to Queue__jki_lib_state_machine.vi"("State(s) in Front (\"\")"="Metadata: Update AI\nMetadata: Update KH\nKH: set KH 0\nKH: set KH 1" ("State(s) in Front (\"\")"), "State(s) in (\"\")"=w213) -> ("States Out"=w215:string)  [unwired: 13 in]
          }
          event Panel Close? {
            n99 = event-data() -> ()  [unwired: 1 in, 1 out]
            n100 = Two Button Dialog(message="Are you sure?") -> (T button?=w221:bool)  [unwired: 2 in]
            n101 = Select(t="Macro: Exit", s=w221, f="") -> (s? t:f=w219:string)
            n102 = event-data ("Event Filter Node")("Discard?"=TRUE) -> ()  [unwired: 1 in, 1 out]
            n103 = call <vilib>:"Add State(s) to Queue__jki_lib_state_machine.vi"("State(s) in Front (\"\")"=w219, "State(s) in (\"\")"=w227) -> ("States Out"=w226:string)  [unwired: 13 in]
          }
        }
      }
      frame "---------- Core ----------" {
        # "Do not put any code in this frame.\n(it is a separator no-op)"
        n104 = call <vilib>:"Add State(s) to Queue__jki_lib_state_machine.vi"("State(s) in (\"\")"=w232) -> ("States Out"=w231:string)  [unwired: 14 in]
      }
      frame Default {
        w243 = 42 items=["No error", "Argument error", "Memory is full", "Out of zone", "End of file", "File already open", "Generic file I/O error", "File not found", "File permission error", "Disk is full", "Duplicate path", "Too many files open", "System feature not enabled", "Resource file not found", "Cannot add resource", "Resource not found", "Image not found", "Image memory error", "Pen does not exist", "Config type invalid", "Config token not found", "Config parse error", "Config memory error", "Bad external code format", "Bad external code offset", "External code not present", "Null window", "Destroy window error", "Null menu", "Print aborted", "Bad print record", "Print driver error", "Windows error during printing", "Memory error during printing", "Print dialog error", "Generic print error", "Invalid device refnum", "Device not found", "Device parameter error", "Device unit error", "Cannot open device", "Device call aborted", "Generic error", "Cancelled by user", "Object ID too low", "Object ID too high", "Object not in heap", "Unknown heap", "Unknown object (invalid DefProc)", "Unknown object (DefProc not in table)", "Message out of range", "Invalid (null) method", "Unknown message", "Manager call not supported", "Bad address", "Network operation in progress", "Network operation timed out", "Connection is busy", "Network attribute not supported", "Network error", "Address in use", "System out of memory", "Connection aborted", "Connection refused", "Not connected", "Already connected", "Connection closed", "Initialization error (interapplication manager)", "Bad occurrence", "Wait on unbound occurrence handler", "Occurrence queue overflow", "Datalog type conflict", "Unused", "Unrecognized type (interapplication manager)", "Memory corrupt", "Failed to make temporary DLL", "Old CIN version", "Drag socket not found", "Failed to load drop-object", "Failed to register OLE object", "Failed to release OLE object", "Format specifier type mismatch", "Unknown format specifier", "Too few format specifiers", "Too many format specifiers", "Scan failed", "Newer CIN version", "Error converting to variant", "Runtime menu error", "Password tampered", "Variant attribute not found", "Incompatible variant data type", "Event data is not available", "Event Store is not present", "Occurrence is not found", "Event Queue is not created", "Event info is not available", "Refnum passed is NULL", "Error retrieving Class GUID", "Error retrieving CoClass GUID", "Error retrieving TypeLib GUID.", "Bad built application magic bytes.", "Specific driver is different from the specific driver associated with the Logical Name.", "There is no session opened to the class driver.", "Max Error", "MAX - Error with config objects", "MAX - Error loading configuration", "MAX - Group not supported"]
        # "Current State"
        # "Handle mistyped state name (developer tool)"
        # "Do not delete, rename, or modify this frame.\n(this is used to capture unhandled states and typos)"
        n105 = Format Into String(format string="Software Exception: Unhandled State \"%s\"." ("message"), error in=w239, w234) -> (resulting string=w242:string, error out=w241:errorcluster)  [unwired: 1 in]
        n106 = call <vilib>:"Error Cluster From Error Code.vi"("show call chain? (False)"=TRUE, "error in (no error)"=w241, "error message (\"\")"=w242, "error code (0)"=w243) -> ("error out"=w240:errorcluster)  [unwired: 5 in]
        n107 = call <vilib>:"Add State(s) to Queue__jki_lib_state_machine.vi"("State(s) in (\"\")"=w238) -> ("States Out"=w237:string)  [unwired: 14 in]
      }
      frame "Initialize Core Data" {
        # "originally closed?"
        # "exe?"
        # "If panel starts closed or is an EXE, then close it when we exit"
        # "Do not delete, rename, or modify this frame.\n(this is used to determine panel behavior on exit)"
        n108 = property on="Property Node" class="VI"() -> ("Front Panel.Open"=w253:bool)  [unwired: 2 in, 2 out]
        n109 = property on="Property Node" class="App"() -> ("App.Kind"=w252:T9)  [unwired: 2 in, 2 out]
        n110 = control-ref of="Current VI Reference"() -> (w246:refnum<vi>)
        n111 = Not(x=w253) -> (.not. x?=w250:bool)
        n112 = Equal?(x=w252, y=T9."Run Time System" ("Application:Kind")) -> (x = y?=w249:bool)
        n113 = Or(x=w250, y=w249) -> (x .or. y?=w247:bool)
        n114 = Bundle By Name(cluster=w248, "Core.Current VI Reference"=w246, "Core.Close Panel on Exit?"=w247) -> (w255:T23)
        n115 = call <vilib>:"Add State(s) to Queue__jki_lib_state_machine.vi"("State(s) in (\"\")"=w257) -> ("States Out"=w256:string)  [unwired: 14 in]
      }
      frame "Error Handler" {
        # "Unhandled Error -- Display it"
        # "Clear error"
        # "Handle any errors here.\nYou can also output any states to clean-up after errors occur"
        n116 = call <vilib>:"General Error Handler.vi"("error in (no error)"=w260) -> ()  [unwired: 10 in, 5 out]
        n117 = call <vilib>:"Add State(s) to Queue__jki_lib_state_machine.vi"("State(s) in Front (\"\")"="/* Post Error States", "State(s) in (\"\")"=w264) -> ("States Out"=w263:string)  [unwired: 13 in]
      }
      frame "Exit" {
        # "Do not put any code in this frame.\n(No errors that occur here will be handled.)"
        n118 = call <vilib>:"Add State(s) to Queue__jki_lib_state_machine.vi"("State(s) in (\"\")"=w270) -> ("States Out"=w269:string)  [unwired: 14 in]
      }
      frame "---------- Data ----------" {
        # "Do not put any code in this frame.\n(It is a separator no-op. You can make a copy of this frame to create a new Data frame)"
        n119 = call <vilib>:"Add State(s) to Queue__jki_lib_state_machine.vi"("State(s) in (\"\")"=w275) -> ("States Out"=w274:string)  [unwired: 14 in]
      }
      frame "Data: Initialize" {
        w278 = refnum<class "Transport.lvclass"> refnum  # Transport
        w277 = refnum<class "Inst.Transport.lvclass"> refnum  # Transport-Server
        w281 = FALSE  # top level?
        w282 = T22 {"Sample"="", "Device"="", "Username"="", "Description"="", "Default Path"=path "", "Instrument"="", "Station Type"="", "KH All Buttons"=enum."No Selection", "Lockin"={"AI"=[], "Electrode"=[], "Label"=[], "Electrode Config"=[], "AI Channels"=16}, "KH"={"KH #"=[], "KH Configuration"=[], "KH Gain"=[], "KH Shunt Resistor"=[], "Filter"=FALSE, "DC Coupled"=FALSE, "KH Chassis"=16}, "non KH"={"Scroll Bar"=[], "Electrodes 2"=[], "Labels 2"=[], "unused"=[]}, "Instrument Types"=[]}  # UI
        w286 = refnum<class "Configuration.lvclass"> refnum  # Config
        w288 = cluster{"Channel Setting":T21}[] []  # Channel Settings
        w284 = T26 {"Current VI Reference"=refnum, "Close Panel on Exit?"=FALSE}  # Core
        # "Initialize the shift-register data, here.\n(data names are defined by what you wire into the bundle function)"
        n120 = Unbundle By Name("C.E.") -> ("Experiment"=w289:T17, "Wiring Configuration"=w290:T20)
        n121 = Bundle("Core"=w284, "C.E."="C.E.", "Experiment"=w289, "Wiring Configuration"=w290, "Channel Settings"=w288, "KH Configuration"="KH Configuration", "Lockin"=w280, "KH"=w279, "non KH"="non KH", "UI"=w282, "Config"=w286, "Transport"=w278, "Transport-Server"=w277, "top level?"=w281) -> (w292:T23)  [unwired: 1 in]
        n122 = call <vilib>:"Add State(s) to Queue__jki_lib_state_machine.vi"("State(s) in (\"\")"=w294) -> ("States Out"=w293:string)  [unwired: 14 in]
      }
      frame "Data: Initialize Top Level" {
        # "Data: Initialize Top Level.\n(Sets top level? == T if Exec.State == Run top level, if not top level, automatically run Macro: Output, Macro: Exit)"
        n123 = property on="Property Node" class="VI"() -> ("Exec.State"=w303:T10)  [unwired: 2 in, 2 out]
        n124 = Equal?(x=w303, y=T10."Run top level" ("Execution:State")) -> (x = y?=w299:bool)
        n125 = Select(t="", s=w299, f="Macro: Output\nMacro: Exit") -> (s? t:f=w298:string)
        n126 = Bundle By Name(cluster=w301, "top level?"=w299) -> (w300:T23)
        n127 = call <vilib>:"Add State(s) to Queue__jki_lib_state_machine.vi"("State(s) in (\"\")"=w306, "State(s) at Back (\"\")"=w298) -> ("States Out"=w305:string)  [unwired: 13 in]
      }
      frame "Data: Load Configuration" {
        # "Data: Load Configuration\n(Load configuration from disk)"
        n128 = Unbundle By Name(w308) -> ("Config"=w317:refnum<class "Configuration.lvclass">, "UI"=w313:T22)
        n129 = call <userlib>:"Default Path.vi"("error in (no error)"=w320, "Folder Name [Application Name]"="Control Experiment" ("name or relative path"), "Configuration in"=w317) -> ("error out"=w315:errorcluster, "Configuration out"=w316:refnum<class "Configuration.lvclass">)  [unwired: 7 in]
        n130 = call <userlib>:"Read Configuration.vi"("INI Fomatted Cluster Type"=w313, "error in (no error)"=w315, "Configuration in"=w316) -> ("error out"=w314:errorcluster, "Configuration"=w311:variant, "Configuration out"=w312:refnum<class "Configuration.lvclass">)  [unwired: 6 in]
        n131 = Variant To Data(error in=w314, type=w313, Variant=w311) -> (data=w309:T22, error out=w319:errorcluster)
        n132 = Bundle By Name(cluster=w308, "Config"=w312, "UI"=w309) -> (w307:T23)
        n133 = call <vilib>:"Add State(s) to Queue__jki_lib_state_machine.vi"("State(s) in (\"\")"=w322) -> ("States Out"=w321:string)  [unwired: 14 in]
      }
      frame "Data: Save Controls" {
        # "Data: Save Controls\n(Write FP controls to UI Cluster and write to disk)"
        n134 = property on="User" class="Ring (strict)"() -> ("RingText.Text"=w327:string)  [unwired: 2 in, 2 out]
        n135 = Unbundle By Name(w334) -> ()  [unwired: 1 out]
        n136 = local read "Sample (SAXXXX)"() -> (w352:string)
        n137 = local read "AI Channels"() -> (w328:u32)
        n138 = local read "Path"() -> (w349:path)
        n139 = local read "KH Configuration"() -> (w348:T7)
        n140 = local read "KH"() -> (w342:T4)
        n141 = local read "Lockin"() -> (w333:T6)
        n142 = local read "non KH"() -> (w343:T8)
        n143 = property on="Station" class="Ring (strict)"() -> ("RingText.Text"=w326:string)  [unwired: 2 in, 2 out]
        n144 = local read "Description"() -> (w350:string)
        n145 = Unbundle By Name(w333) -> ("AI"=w332:u32[], "Electrode"=w331:string[], "Label"=w330:u16[], "Electrode Config"=w329:T5[])
        n146 = local read "Device"() -> (w351:string)
        n147 = Unbundle By Name(w342) -> ("KH #"=w341:u16[], "KH Configuration"=w338:T1[], "KH Gain"=w339:T2[], "KH Shunt Resistor"=w340:T3[])
        n148 = property on="Type" class="Ring (strict)"() -> ("RingText.Text"=w325:string)  [unwired: 2 in, 2 out]
        n149 = local read "KH Chassis"() -> (w324:i32)
        n150 = Bundle By Name(cluster=w334, "UI.Sample"=w352, "UI.Device"=w351, "UI.Username"=w327, "UI.Description"=w350, "UI.Default Path"=w349, "UI.Instrument"=w326, "UI.Station Type"=w325, "UI.KH All Buttons"=w348, "UI.Lockin.AI"=w332, "UI.Lockin.Electrode"=w331, "UI.Lockin.Label"=w330, "UI.Lockin.Electrode Config"=w329, "UI.Lockin.AI Channels"=w328, "UI.non KH"=w343, "UI.KH.KH #"=w341, "UI.KH.KH Configuration"=w338, "UI.KH.KH Gain"=w339, "UI.KH.KH Shunt Resistor"=w340, "UI.KH.Filter"="BW Filter", "UI.KH.DC Coupled"="DC Coupled", "UI.KH.KH Chassis"=w324) -> (w335:T23)
        n151 = Unbundle By Name(w335) -> ("Config"=w347:refnum<class "Configuration.lvclass">, "UI"=w346:T22)
        n152 = call <userlib>:"Write Configuration.vi"("error in (no error)"=w345, "Variant"=w346, "Configuration in"=w347) -> ("error out"=w344:errorcluster)  [unwired: 7 in, 1 out]
        n153 = call <vilib>:"Add State(s) to Queue__jki_lib_state_machine.vi"("State(s) in (\"\")"=w354) -> ("States Out"=w353:string)  [unwired: 14 in]
      }
      frame "Data: Cleanup" {
        # "Cleanup any data and references, here.\n(this is called automatically, by the Macro: Exit)"
        n154 = Unbundle By Name(w358) -> ("Core.Current VI Reference"=w357:refnum<vi>)
        n155 = Close Reference(reference=w357, error in (no error)=w356) -> (error out=w359:errorcluster)
        n156 = call <vilib>:"Add State(s) to Queue__jki_lib_state_machine.vi"("State(s) in (\"\")"=w361) -> ("States Out"=w360:string)  [unwired: 14 in]
      }
      frame "Data: Query Database" {
        # "Do not put any code in this frame.\n(It is a separator no-op. You can make a copy of this frame to create a new Data frame)"
        n157 = Unbundle By Name(w383) -> ("UI.Station Type"=w375:string, "UI.Instrument"=w367:string, "UI.Username"=w385:string)
        n158 = call "DB Get Station Type.vi"() -> ("Station Types"=w374:string[])  [unwired: 10 in, 1 out]
        n159 = Search 1D Array(1D array=w374, element=w375) -> (index of element=w376:i32)  [unwired: 1 in]
        n160 = property on="Type" class="Ring (strict)"("Strings []"=w374) -> (error out=w373:errorcluster)  [unwired: 2 in, 1 out]
        n161 = call "DB Get Current Users.vi"() -> ("Result (Rows or Columns)"=w379:string[])  [unwired: 10 in, 1 out]
        n162 = Less Than 0?(x=w376) -> (x < 0?=w378:bool)
        n163 = Select(t=0, s=w378, f=w376) -> (s? t:f=w372:i32)
        n164 = property on="User" class="Ring (strict)"("Strings []"=w379) -> ()  [unwired: 2 in, 2 out]
        n165 = property on="Type" class="Ring (strict)"(error in=w373, "Value"=w372) -> (error out=w371:errorcluster)  [unwired: 1 in, 1 out]
        n166 = property on="Type" class="Ring (strict)"(error in=w371) -> ("RingText.Text"=w363:string)  [unwired: 1 in, 2 out]
        n167 = Search 1D Array(1D array=w379, element=w385) -> (index of element=w388:i32)  [unwired: 1 in]
        n168 = Less Than 0?(x=w388) -> (x < 0?=w386:bool)
        n169 = Select(t=0, s=w386, f=w388) -> (s? t:f=w381:i32)
        n170 = call "DB Get Stations.vi"("Station Type"=w363) -> ("Stations"=w366:string[])  [unwired: 9 in, 1 out]
        n171 = property on="User" class="Ring (strict)"("Value"=w381) -> ("Strings []"=w382:string[])  [unwired: 2 in, 2 out]
        n172 = property on="Station" class="Ring (strict)"("Strings []"=w366) -> ()  [unwired: 2 in, 2 out]
        n173 = Search 1D Array(1D array=w366, element=w367) -> (index of element=w368:i32)  [unwired: 1 in]
        n174 = Index Array(array=w382, index=w381) -> (element=w380:string)
        n175 = Less Than 0?(x=w368) -> (x < 0?=w370:bool)
        n176 = Select(t=0, s=w370, f=w368) -> (s? t:f=w365:i32)
        n177 = property on="Station" class="Ring (strict)"("Strings []"=w366, "Value"=w365) -> ()  [unwired: 2 in, 2 out]
        n178 = Index Array(array=w366, index=w365) -> (element=w364:string)
        n179 = Bundle By Name(cluster=w383, "UI.Instrument"=w364, "UI.Station Type"=w363, "UI.Username"=w380) -> (w384:T23)
        n180 = call <vilib>:"Add State(s) to Queue__jki_lib_state_machine.vi"("State(s) in (\"\")"=w391) -> ("States Out"=w390:string)  [unwired: 14 in]
      }
      frame "---------- Events ----------" {
        # "Do not put any code in this frame.\n(It is a separator no-op. You can make a copy of this frame to create a new UI frame)"
        n181 = call <vilib>:"Add State(s) to Queue__jki_lib_state_machine.vi"("State(s) in (\"\")"=w396) -> ("States Out"=w395:string)  [unwired: 14 in]
      }
      frame "Events: Register" {
        # "Do not put any code in this frame.\n(It is a separator no-op. You can make a copy of this frame to create a new UI frame)"
        n182 = Unbundle By Name(w407) -> ("Transport-Server"=w406:refnum<class "Inst.Transport.lvclass">)
        n183 = call <vilib>:"GetPublicEvents.vi"("SMO"=w406) -> ("error out"=w397:errorcluster, "Public Events"=w405:T27, "SMO out"=w400:refnum<class "Inst.Transport.lvclass">)  [unwired: 8 in]
        n184 = call "Inst.Transport.GetPublicEvents.vi"("Inst.Transport in"=w400) -> ("error out"=w398:errorcluster, "Transport Public Events"=w399:T28)  [unwired: 8 in, 1 out]
        n185 = register-events(w405, w399) -> (reference out=w401:refnum<event-registration>, error out=w404:errorcluster)  [unwired: 2 in]
        n186 = Merge Errors(w404, w398, w397, w402) -> (w403:errorcluster)
        n187 = call <vilib>:"Add State(s) to Queue__jki_lib_state_machine.vi"("State(s) in (\"\")"=w409) -> ("States Out"=w408:string)  [unwired: 14 in]
      }
      frame "Events: Unregister" {
        # "Do not put any code in this frame.\n(It is a separator no-op. You can make a copy of this frame to create a new UI frame)"
        n188 = Unregister For Events(event registration refnum=w412, error in=w411) -> (error out=w410:errorcluster)
        n189 = call <vilib>:"Add State(s) to Queue__jki_lib_state_machine.vi"("State(s) in (\"\")"=w415) -> ("States Out"=w414:string)  [unwired: 14 in]
      }
      frame "---------- UI ----------" {
        # "Do not put any code in this frame.\n(It is a separator no-op. You can make a copy of this frame to create a new UI frame)"
        n190 = call <vilib>:"Add State(s) to Queue__jki_lib_state_machine.vi"("State(s) in (\"\")"=w420) -> ("States Out"=w419:string)  [unwired: 14 in]
      }
      frame "UI: Initialize" {
        w421 = "" ("MCL S/N")
        w431 = FALSE ("KH?")
        # "Initialize the User Interface, here.\n(this is called automatically, by the Macro: Init)"
        n191 = call <userlib>:"Fit VI window to Largest Dec__ogtk.vi"("error in (no error)"=w440, "border spacing (2 px)"=0) -> ("error out"=w424:errorcluster)  [unwired: 4 in, 1 out]
        n192 = Unbundle By Name(w435) -> ("top level?"=w434:bool)
        n193 = property on="OK" class="Bool (strict)"("Value"=FALSE ("Blinking")) -> ()  [unwired: 2 in, 2 out]
        n194 = property on="Tab Control" class="TabCtl (strict)"("Value"=enum32{"Input", "Output", "Configuration"}."Input" ("Tab Control")) -> ()  [unwired: 2 in, 2 out]
        n195 = local write "KH Configuration"(T7."No Selection" ("KH All Buttons")) -> ()
        n196 = property on="Values have changed" class="Bool (strict)"("Val(Sgnl)"=TRUE ("Blinking")) -> ()  [unwired: 2 in, 2 out]
        n197 = call <vilib>:"1D String Array to Delimited String.vi"("delimiter"="\n", "string array"=string[] ["", "I+", "I-", "V1+", "V1-", "V2+", "V2-", "V3+", "V3-", "V4+", "V4-", "dV1", "dV2", "dV3", "Vsg", "Vbg", "Vtg"] ("Strings [] 2")) -> ("delimited string"=w425:string)  [unwired: 9 in]
        n198 = local write "MCL S/N"(w421) -> ()
        n199 = local write "KH S/N"(w421) -> ()
        n200 = local write "Label Strings"(w425) -> ()
        n201 = case shown="True" w434 {
          frame False {
          }
          frame True {
            # "unused"
            n202 = property on="AI Channels" class="DigNum (strict)"("Val(Sgnl)"="AI Channels") -> ()  [unwired: 2 in, 2 out]
          }
        }
        n203 = call <vilib>:"Delimited String to 1D String Array.vi"("delimiter"="\n", "delimited string"=w425) -> ("string array"=w429:string[])  [unwired: 9 in]
        n204 = property on="Ring" class="Ring (strict)"("Strings []"=w429) -> (error out=w438:errorcluster)  [unwired: 2 in, 1 out]
        n205 = local write "Transport Server"(w431) -> ()
        n206 = property on="Ring" class="Ring (strict)"(error in=w438, "Strings []"=w429) -> (error out=w422:errorcluster)  [unwired: 1 in, 1 out]
        n207 = Merge Errors(w422, w424) -> (w423:errorcluster)
        n208 = call <vilib>:"Add State(s) to Queue__jki_lib_state_machine.vi"("State(s) in (\"\")"=w442) -> ("States Out"=w441:string)  [unwired: 14 in]
        "Lockin?" <- w431
        "KH?" <- w431
        "Transport?" <- w431
      }
      frame "UI: Update Controls" {
        # "UI: Update Controls\n(Update FP from UI cluster)"
        n209 = Unbundle By Name(w462) -> ("top level?"=w463:bool, "UI.Sample"=w467:string, "UI.Device"=w468:string, "UI.Description"=w469:string, "UI.Default Path"=w470:path, "UI.KH All Buttons"=w466:T7, "UI.Lockin"=w453:T29, "UI.KH"=w446:T30, "UI.non KH"=w457:T8)  [unwired: 2 out]
        n210 = local write "KH Configuration"(w466) -> ()
        n211 = local write "Sample (SAXXXX)"(w467) -> ()
        n212 = local write "Path"(w470) -> ()
        n213 = Unbundle By Name(w453) -> ("AI"=w452:u32[], "Electrode"=w448:string[], "Label"=w449:u16[], "Electrode Config"=w450:T5[], "AI Channels"=w447:u32)
        n214 = Unbundle By Name(w446) -> ("KH #"=w461:T31, "KH Configuration"=w458:T1[], "KH Gain"=w459:T2[], "KH Shunt Resistor"=w460:T3[], "Filter"=w456:bool, "DC Coupled"=w455:bool, "KH Chassis"=w445:i32)
        n215 = local write "Description"(w469) -> ()
        n216 = local write "Device"(w468) -> ()
        n217 = local read "Lockin"() -> (w454:T6)
        n218 = Bundle By Name(cluster=w454, "AI"=w452, "Electrode"=w448, "Label"=w449, "Electrode Config"=w450) -> (w451:T6)
        n219 = local read "KH"() -> (w465:T4)
        n220 = Bundle By Name(cluster=w465, "KH #"=w461, "KH Configuration"=w458, "KH Gain"=w459, "KH Shunt Resistor"=w460) -> (w464:T4)
        n221 = case shown="True" w463 {
          tunnel: w464 -> [_ w480]
          tunnel: w457 -> [_ w479]
          tunnel: w456 -> [_ w478]
          tunnel: w455 -> [_ w477]
          tunnel: w451 -> [_ w476]
          tunnel: w447 -> [_ w475]
          tunnel: w445 -> [_ w474]
          frame False {
          }
          frame True {
            n222 = local write "Lockin"(w476) -> ()
            n223 = local write "AI Channels"(w475) -> ()
            n224 = local write "KH"(w480) -> ()
            n225 = local write "DC Coupled"(w477) -> ()
            n226 = local write "non KH"(w479) -> ()
            n227 = local write "KH Chassis"(w474) -> ()
            n228 = local write "BW Filter"(w478) -> ()
          }
        }
        n229 = call <vilib>:"Add State(s) to Queue__jki_lib_state_machine.vi"("State(s) in (\"\")"=w473) -> ("States Out"=w472:string)  [unwired: 14 in]
      }
      frame "UI: View Instruments" {
        # "UI: View Instruments\n(convert Experiment.Instrument array to string)"
        n230 = Unbundle By Name(w491) -> ("C.E."=w482:refnum<class "Control Experiment.lvclass">)
        n231 = Cluster To Array(cluster=T11 {"DAQ"=refnum, "Amplifier"=refnum, "Temperature"=refnum, "Magnet"=refnum, "Rotator"=refnum, "Level"=refnum, "Capacitance"=refnum, "Delay Line"=refnum, "Strain Cell"=refnum, "VNA"=refnum, "Source"=refnum} ("Instrument Classes")) -> (array=w483:refnum<class "Instrument.lvclass">[])
        n232 = Unbundle By Name(w482) -> ("Instruments"=w490:T18[])
        n233 = for {
          tunnel: w483 -> [w499] mode=indexing
          tunnel: [w496] -> w481 mode=indexing
          tunnel: [w494] -> _
          n234 = call <vilib>:"Get LV Class Name.vi"("object"=w499) -> ("error out"=w495:errorcluster, "class name"=w497:string)  [unwired: 9 in]
          n235 = String To Path(string=w497) -> (path=w498:path)
          n236 = call <vilib>:"Get File Extension.vi"("error in (no error)"=w495, "file"=w498) -> ("error out"=w494:errorcluster, "filename without extension"=w496:string)  [unwired: 5 in, 3 out]
        }
        n237 = for {
          tunnel: w490 -> [w508] mode=indexing
          tunnel: [w506] -> w489 mode=indexing
          tunnel: w481 -> [w504]
          n238 = Unbundle By Name(w508) -> ("Type"=w507:T19, "class path"=w505:path, "Address"=w503:string)
          n239 = call <vilib>:"Get File Extension.vi"("file"=w505) -> ("filename without extension"=w501:string)  [unwired: 6 in, 4 out]
          n240 = call <vilib>:"Parse URI.vi"("URI"=w503) -> ("address"=w500:string)  [unwired: 6 in, 4 out]
          n241 = call <userlib>:"MGI String Pattern Match Exists.vi"("Patterns to Try"=w504, "String"=w501) -> ("Match Found"=w502:bool)  [unwired: 1 out]
          n242 = case shown="False" w502 {
            tunnel: w507 -> [w512 _]
            tunnel: [w511 ""] -> w506
            tunnel: w500 -> [w510 _]
            tunnel: w501 -> [w509 _]
            frame False {
              n243 = case shown="\"\"" w510 {
                selector: w510 -> [w513 _]
                tunnel: w512 -> [w516 w520]
                tunnel: w509 -> [w515 w519]
                tunnel: [w514 w518] -> w511
                frame Default {
                  n244 = Format Into String(format string="- %s: %s\n   - %s", w516, w515, w513) -> (resulting string=w514:string)  [unwired: 2 in, 1 out]
                }
                frame "" {
                  n245 = Format Into String(format string="- %s: %s", w520, w519) -> (resulting string=w518:string)  [unwired: 2 in, 1 out]
                }
              }
            }
            frame True {
            }
          }
        }
        n246 = call <vilib>:"1D String Array to Delimited String.vi"("delimiter"="\n", "string array"=w489) -> ("delimited string"=→"Configured Instruments":string)  [unwired: 9 in]
        n247 = call <vilib>:"Add State(s) to Queue__jki_lib_state_machine.vi"("State(s) in (\"\")"=w493) -> ("States Out"=w492:string)  [unwired: 14 in]
      }
      frame "UI: Cursor Set" {
        # "Argument"
        # "Set and Unset Cursor Busy.\n(Usage: \"UI: Cursor Set >> Busy|Idle\")"
        n248 = case shown="\"Idle\", Default" w524 {
          tunnel: w526 -> [w531 w533]
          tunnel: [w530 w532] -> w525
          frame "Idle", Default {
            n249 = call <vilib>:"Unset Busy.vi"("error in (no error)"=w531) -> ("error out"=w530:errorcluster)  [unwired: 10 in]
          }
          frame "Busy" {
            n250 = call <vilib>:"Set Busy.vi"("error in (no error)"=w533) -> ("error out"=w532:errorcluster)  [unwired: 9 in, 1 out]
          }
        }
        n251 = call <vilib>:"Add State(s) to Queue__jki_lib_state_machine.vi"("State(s) in (\"\")"=w529) -> ("States Out"=w528:string)  [unwired: 14 in]
      }
      frame "UI: Front Panel State" {
        # "Argument"
        # "Set Front Panel Open or Closed\n(Usage: \"UI: Front Panel State >> Open|Close\")"
        n252 = Unbundle By Name(w537) -> ("Core.Current VI Reference"=w536:refnum<vi>)
        n253 = case shown="\"Open\", Default" w535 {
          tunnel: w539 -> [w545 w558]
          tunnel: [w547 w559] -> w538
          tunnel: w536 -> [w546 w556]
          frame "Open", Default {
            n254 = property on="Property Node" class="VI"(reference=w546, error in=w545) -> (reference out=w543:refnum<vi>, error out=w544:errorcluster, "Front Panel.Open"=w542:bool)
            n255 = case shown="True" w542 {
              tunnel: [w550 w553] -> w547
              tunnel: w544 -> [w549 w553]
              tunnel: w543 -> [w548 _]
              frame False {
                n256 = invoke on="Invoke Node" class="VI" method="FP.Open"(reference=w548, error in=w549, "Activate"=TRUE, "State"=T12."Standard") -> (error out=w550:errorcluster)  [unwired: 1 in, 4 out]
              }
              frame True {
              }
            }
          }
          frame "Close" {
            n257 = property on="Property Node" class="VI"(reference=w556, error in=w558) -> (reference out=w555:refnum<vi>, error out=w557:errorcluster, "Front Panel.Open"=w554:bool)
            n258 = case shown="True" w554 {
              tunnel: [w560 w563] -> w559
              tunnel: w557 -> [w560 w562]
              tunnel: w555 -> [_ w561]
              frame False {
              }
              frame True {
                n259 = invoke on="Invoke Node" class="VI" method="FP.Close"(reference=w561, error in=w562) -> (error out=w563:errorcluster)  [unwired: 1 in, 2 out]
              }
            }
          }
        }
        n260 = call <vilib>:"Add State(s) to Queue__jki_lib_state_machine.vi"("State(s) in (\"\")"=w541) -> ("States Out"=w540:string)  [unwired: 14 in]
      }
      frame "UI: Buttons" {
        # "UI: Buttons"
        n261 = call <vilib>:"Add State(s) to Queue__jki_lib_state_machine.vi"("State(s) in (\"\")"=w568) -> ("States Out"=w567:string)  [unwired: 14 in]
      }
      frame "UI: Link Scroll Bars" {
        # "UI: Link Scroll Bars\n(Link all scroll bars of control arrays)"
        n262 = control-ref of="AI"() -> (w580:refnum<vi>)
        n263 = control-ref of="Electrode"() -> (w579:refnum<vi>)
        n264 = control-ref of="Label"() -> (w578:refnum<vi>)
        n265 = control-ref of="Electrode Config"() -> (w577:refnum<vi>)
        n266 = control-ref of="KH #"() -> (w576:refnum<vi>)
        n267 = control-ref of="KH Configuration"() -> (w575:refnum<vi>)
        n268 = control-ref of="KH Gain"() -> (w574:refnum<vi>)
        n269 = control-ref of="KH Shunt Resistor"() -> (w573:refnum<vi>)
        n270 = control-ref of="Gain"() -> (w571:refnum<vi>)
        n271 = property on="Property Node" class="Arr (strict)"(reference=w580) -> ("Index Values"=w570:u32[])  [unwired: 1 in, 2 out]
        n272 = property on="Property Node" class="Arr (strict)"(reference=w579, "Index Values"=w570) -> ()  [unwired: 1 in, 2 out]
        n273 = property on="Property Node" class="Arr (strict)"(reference=w578, "Index Values"=w570) -> ()  [unwired: 1 in, 2 out]
        n274 = property on="Property Node" class="Arr (strict)"(reference=w577, "Index Values"=w570) -> ()  [unwired: 1 in, 2 out]
        n275 = property on="Property Node" class="Arr (strict)"(reference=w576, "Index Values"=w570) -> ()  [unwired: 1 in, 2 out]
        n276 = property on="Property Node" class="Arr (strict)"(reference=w575, "Index Values"=w570) -> ()  [unwired: 1 in, 2 out]
        n277 = property on="Property Node" class="Arr (strict)"(reference=w574, "Index Values"=w570) -> ()  [unwired: 1 in, 2 out]
        n278 = property on="Property Node" class="Arr (strict)"(reference=w573, "Index Values"=w570) -> ()  [unwired: 1 in, 2 out]
        n279 = property on="Property Node" class="Arr (strict)"(reference=w571, "Index Values"=w570) -> ()  [unwired: 1 in, 2 out]
        n280 = property on="Scroll Bar" class="Arr (strict)"() -> ("Index Values"=w572:u32[])  [unwired: 2 in, 2 out]
        n281 = property on="Labels 2" class="Arr (strict)"("Index Values"=w572) -> ()  [unwired: 2 in, 2 out]
        n282 = property on="unused" class="Arr (strict)"("Index Values"=w572) -> ()  [unwired: 2 in, 2 out]
        n283 = property on="Electrodes 2" class="Arr (strict)"("Index Values"=w572) -> ()  [unwired: 2 in, 2 out]
        n284 = call <vilib>:"Add State(s) to Queue__jki_lib_state_machine.vi"("State(s) in (\"\")"=w584) -> ("States Out"=w583:string)  [unwired: 14 in]
      }
      frame "UI: SR Disable" {
        # "UI: SR Disable\n(Checks if attached KH7008 is configured with 500 or 10M shunt resistor)"
        n285 = Unbundle By Name(w597) -> ("C.E."=w592:refnum<class "Control Experiment.lvclass">)
        n286 = Unbundle By Name(w592) -> ("Amplifier"=w594:refnum<class "Instrument.Amplifier.lvclass">)
        n287 = local read "KH Chassis"() -> (w585:i32)
        n288 = To More Specific Class(target class=refnum<class "Inst.Krohn-Hite-7008.lvclass"> refnum ("Inst.KH7008.lvlib:Inst.Krohn-Hite-7008.lvclass"), reference=w594) -> (specific class reference=w593:refnum<class "Inst.Krohn-Hite-7008.lvclass">)  [unwired: 1 in, 1 out]
        n289 = for {
          N: w585 -> [_]
          tunnel: w593 -> [w610]
          tunnel: [w603] -> w591 mode=concatenating
          tunnel: w590 -> [w600]
          tunnel: [w611] -> w589
          i -> [w602]
          # "check"
          # "disable"
          n290 = Increment(x=w602) -> (x+1=w601:i32)
          n291 = call-dynamic "Inst.KH7008.Open.vi"("error in (no error)"=w600, "index"=w601, "Inst.Krohn-Hite-7008 in"=w610) -> ("error out"=w607:errorcluster, "Inst.Krohn-Hite-7008 out"=w609:refnum<class "Inst.Krohn-Hite-7008.lvclass">)  [unwired: 7 in]
          n292 = call-dynamic "Inst.KH7008.getShuntResistor.vi"("error in (no error)"=w607, "Inst.Krohn-Hite-7008 in"=w609) -> ("error out"=w606:errorcluster, "ShuntResistor"=w605:string, "Inst.Krohn-Hite-7008 out"=w608:refnum<class "Inst.Krohn-Hite-7008.lvclass">)  [unwired: 7 in]
          n293 = case shown="Default" w605 {
            tunnel: [2 5] -> w604
            frame Default {
            }
            frame "500" {
            }
          }
          n294 = call-dynamic "Close.vi"("error in (no error)"=w606, "Inst.Krohn-Hite-7008 in"=w608) -> ("error out"=w611:errorcluster)  [unwired: 8 in, 1 out]
          n295 = Build Array(w604) -> (w603:i32[])
        }
        n296 = control-ref of="Shunt Resistor"() -> (w587:refnum<vi>)
        n297 = control-ref of="Default Resistor"() -> (w588:refnum<vi>)
        n298 = Build Array(w587, w588) -> (w586:refnum<vi>[])
        n299 = for {
          tunnel: w591 -> [w615]
          tunnel: w586 -> [w614] mode=indexing
          # "disable"
          n300 = property on="Property Node" class="Enum (strict)"(reference=w614, "Disabled Items []"=w615) -> ()  [unwired: 1 in, 2 out]
        }
        n301 = call <vilib>:"Add State(s) to Queue__jki_lib_state_machine.vi"("State(s) in (\"\")"=w599) -> ("States Out"=w598:string)  [unwired: 14 in]
      }
      frame "---------- Macro ----------" {
        # "Do not put any code in this frame.\n(It is a separator no-op. You can make a copy of this frame to create a new Macro frame)"
        n302 = call <vilib>:"Add State(s) to Queue__jki_lib_state_machine.vi"("State(s) in (\"\")"=w620) -> ("States Out"=w619:string)  [unwired: 14 in]
      }
      frame "Macro: Initialize" {
        # "Instruments: Load Classes\nUI: View Instruments\nMetadata: Write FGV"
        # "Initialization Macro\n(This is called once, when the VI starts)"
        n303 = call <vilib>:"Add State(s) to Queue__jki_lib_state_machine.vi"("State(s) in Front (\"\")"="Data: Initialize\nInitialize Core Data\nUI: Initialize\nUI: Front Panel State >> Open\nTransport Server: Create\nEvents: Register\nTransport Server: Start\nData: Initialize Top Level\nData: Load Configuration\nMetadata: Read FGV\n\nUI: Update Controls\n\nUI: View Instruments\nUI: Update Controls\nData: Query Database\n\nInstrument: Lockin Status\nInstrument: KH Status", "State(s) in (\"\")"=w626) -> ("States Out"=w625:string)  [unwired: 13 in]
      }
      frame "Macro: Exit" {
        # "Exit Macro\n(This is called once, when the VI exits)"
        n304 = Unbundle By Name(w635) -> ("Core.Close Panel on Exit?"=w634:bool)
        n305 = property on="OK" class="Bool (strict)"("Value"=FALSE ("Blinking")) -> ()  [unwired: 2 in, 2 out]
        n306 = Select(t="UI: Front Panel State >> Close", s=w634, f="" ("Empty String Constant")) -> (s? t:f=w631:string)
        n307 = call <vilib>:"Add State(s) to Queue__jki_lib_state_machine.vi"("State(s) in (\"\")"=w631, "State(s) at Back (\"\")"="Data: Save Controls\nTransport Server: Stop\nTransport Server: Destroy\nData: Cleanup\nEvents: Unregister\nExit") -> ("States Out"=w629:string)  [unwired: 13 in]
        n308 = call <vilib>:"Add State(s) to Queue__jki_lib_state_machine.vi"("State(s) in Front (\"\")"=w629, "State(s) in (\"\")"=w638) -> ("States Out"=w637:string)  [unwired: 13 in]
      }
      frame "Macro: Output" {
        # "Macro: Output\n(Set KH7008, Write Metadata to FGV.JSON, Write Metadata to PGSQL (Device and User))"
        n309 = case shown="False" "I'm Finished Taking Data!" {
          tunnel: ["Macro: Initialize Metadata\nUI: SR Disable\nKH: set KH 0\nKH: set KH 1\nKH: set KH 2\nMacro: Write Metadata" ("State(s) in Front (\"\")") _] -> w643
          frame False {
          }
          frame True {
          }
        }
        n310 = call <vilib>:"Add State(s) to Queue__jki_lib_state_machine.vi"("State(s) in Front (\"\")"=w643, "State(s) in (\"\")"=w646, "State(s) at Back (\"\")"="PGSQL: Write" ("State(s) in Front (\"\")")) -> ("States Out"=w645:string)  [unwired: 12 in]
      }
      frame "Macro: Instrument Configuration Changed" {
        # "Do not put any code in this frame.\n(It is a separator no-op. You can make a copy of this frame to create a new Macro frame)"
        n311 = call <vilib>:"Add State(s) to Queue__jki_lib_state_machine.vi"("State(s) in Front (\"\")"="Instruments: Load Classes\nUI: View Instruments\nMetadata: Write FGV\nInstrument: Lockin Status\nInstrument: KH Status" ("State(s) in Front (\"\")"), "State(s) in (\"\")"=w653) -> ("States Out"=w652:string)  [unwired: 13 in]
      }
      frame "Macro: Initialize Metadata" {
        # "Macro: Initialize Metadata"
        n312 = call <vilib>:"Add State(s) to Queue__jki_lib_state_machine.vi"("State(s) in Front (\"\")"="Metadata: Update Experiment Description\nMetadata: Update Wiring Configuration\nMetadata: Update KH\nMetadata: Build Path\nMetadata: Update Control Experiment Wire" ("State(s) in Front (\"\")"), "State(s) in (\"\")"=w659) -> ("States Out"=w658:string)  [unwired: 13 in]
      }
      frame "Macro: Write Metadata" {
        # "Macro: Write Metadata"
        n313 = call <vilib>:"Add State(s) to Queue__jki_lib_state_machine.vi"("State(s) in Front (\"\")"="Metadata: Update Comments\nMetadata: Write JSON\nMetadata: Write FGV" ("State(s) in Front (\"\")"), "State(s) in (\"\")"=w665) -> ("States Out"=w664:string)  [unwired: 13 in]
      }
      frame "---------- Metadata ----------" {
        # "Do not put any code in this frame.\n(it is a separator no-op)"
        n314 = call <vilib>:"Add State(s) to Queue__jki_lib_state_machine.vi"("State(s) in (\"\")"=w670) -> ("States Out"=w669:string)  [unwired: 14 in]
      }
      frame "Metadata: Update Experiment Description" {
        n315 = property on="Station" class="Ring (strict)"() -> ("RingText.Text"=w672:string)  [unwired: 2 in, 2 out]
        n316 = property on="User" class="Ring (strict)"() -> ("RingText.Text"=w673:string)  [unwired: 2 in, 2 out]
        n317 = Concatenate Strings("Sample (SAXXXX)", "." ("string"), "Device") -> (w675:string)
        n318 = Bundle By Name(cluster=w679, "Experiment.Device"=w675, "Experiment.Device Description"="Description", "Experiment.User"=w673, "Experiment.Instrument"=w672) -> (w680:T23)
        n319 = call <vilib>:"Add State(s) to Queue__jki_lib_state_machine.vi"("State(s) in (\"\")"=w683) -> ("States Out"=w682:string)  [unwired: 14 in]
      }
      frame "Metadata: Update Wiring Configuration" {
        n320 = local read "Lockin"() -> (w695:T6)
        n321 = local read "non KH"() -> (w689:T8)
        n322 = local read "Lockin"() -> (w693:T6)
        n323 = Unbundle By Name(w689) -> ("Electrodes 2"=w688:string[], "Labels 2"=w687:u16[])
        n324 = Unbundle By Name(w695) -> ("AI"=w690:u32[], "Electrode"=w691:string[], "Label"=w694:u16[])
        n325 = Unbundle By Name(w693) -> ("Electrode Config"=w692:T5[])
        n326 = To Long Integer(number=w687) -> (32bit integer=w684:i32[])
        n327 = To Long Integer(number=w694) -> (32bit integer=w685:i32[])
        n328 = for {
          tunnel: w684 -> [w704] mode=indexing
          tunnel: [w703] -> w696 mode=indexing
          n329 = property on="Ring" class="Ring (strict)"() -> ("Strings []"=w705:string[])  [unwired: 2 in, 2 out]
          n330 = Index Array(array=w705, index=w704) -> (element=w703:string)
        }
        n331 = for {
          tunnel: w685 -> [w707] mode=indexing
          tunnel: [w706] -> w697 mode=indexing
          n332 = property on="Ring" class="Ring (strict)"() -> ("Strings []"=w708:string[])  [unwired: 2 in, 2 out]
          n333 = Index Array(array=w708, index=w707) -> (element=w706:string)
        }
        n334 = Bundle By Name(cluster=w698, "Wiring Configuration.Lockin Ch"=w690, "Wiring Configuration.KH.Electrodes"=w691, "Wiring Configuration.KH.Labels"=w697, "Wiring Configuration.not KH.Electrodes"=w688, "Wiring Configuration.not KH.Labels"=w696, "Lockin.Electrode Config"=w692) -> (w699:T23)
        n335 = call <vilib>:"Add State(s) to Queue__jki_lib_state_machine.vi"("State(s) in (\"\")"=w702) -> ("States Out"=w701:string)  [unwired: 14 in]
      }
      frame "Metadata: Update KH" {
        n336 = local read "KH"() -> (w724:T4)
        n337 = Unbundle By Name(w724) -> ("KH Gain"=w716:T2[], "KH Configuration"=w721:T1[], "KH Shunt Resistor"=w720:T3[], "KH #"=w713:u16[])
        n338 = Empty Array?(array=w713) -> (empty?=w714:bool)
        n339 = case shown="False" w714 {
          tunnel: [w737 w768] -> w723
          tunnel: w721 -> [w736 _]
          tunnel: w720 -> [w735 _]
          tunnel: [w734 w766] -> w719
          tunnel: w713 -> [w730 _]
          tunnel: [w733 w769] -> w718
          tunnel: [w732 w767] -> w717
          tunnel: w716 -> [w729 _]
          tunnel: w715 -> [w731 w769]
          tunnel: [w730 u16[] [] ("KH #")] -> w712
          frame False {
            n340 = Empty Array?(array=w729) -> (empty?=w728:bool)
            n341 = case shown="False" w728 {
              tunnel: [w752 w756] -> w737
              tunnel: w736 -> [w748 w758]
              tunnel: w735 -> [w747 w759]
              tunnel: [w746 w754] -> w734
              tunnel: [w745 w753] -> w733
              tunnel: [w744 w755] -> w732
              tunnel: w731 -> [w743 w753]
              tunnel: w729 -> [w739 w757]
              tunnel: w730 -> [w738 w760]
              frame False {
                n342 = call "Initialize KH Array.vi"("KH #"=w738, "Control in"=w739) -> ("Control out"=w751:variant)  [unwired: 9 in]
                n343 = call "Initialize KH Array.vi"("KH #"=w738, "Control in"=w748) -> ("Control out"=w750:variant)  [unwired: 9 in]
                n344 = call "Initialize KH Array.vi"("KH #"=w738, "Control in"=w747) -> ("Control out"=w749:variant)  [unwired: 9 in]
                n345 = Variant To Data(error in=w743, type=w739, Variant=w751) -> (data=w752:T2[], error out=w742:errorcluster)
                n346 = Variant To Data(error in=w743, type=w748, Variant=w750) -> (data=w744:T1[], error out=w741:errorcluster)
                n347 = Variant To Data(error in=w743, type=w747, Variant=w749) -> (data=w746:T3[], error out=w740:errorcluster)
                n348 = Merge Errors(w742, w741, w740) -> (w745:errorcluster)
              }
              frame True {
                n349 = Array Size(array=w760) -> (size(s)=w761:i32)
                n350 = Index Array(array=w758) -> (element=w763:T1)  [unwired: 1 in]
                n351 = Index Array(array=w759) -> (element=w762:T3)  [unwired: 1 in]
                n352 = Index Array(array=w757) -> (element=w764:T2)  [unwired: 1 in]
                n353 = Initialize Array(w764, w761) -> (w756:T2[])
                n354 = Initialize Array(w763, w761) -> (w755:T1[])
                n355 = Initialize Array(w762, w761) -> (w754:T3[])
              }
            }
          }
          frame True {
            w766 = T3[] [] items=["Open", "50", "500", "5k", "50k", "10M"] ("KH Shunt Resistor")
            w767 = T1[] [] items=["OFF", "SE+", "SE-", "DIFF"] ("KH Configuration")
            w768 = T2[] [] items=["1", "10", "100", "1000"] ("KH Gain")
          }
        }
        n356 = local read "KH Configuration"() -> (w722:T7)
        n357 = Bundle By Name(cluster=w725, "KH Configuration"=w722, "KH.KH Gain"=w723, "KH.KH Configuration"=w717, "KH.KH Shunt Resistor"=w719, "KH.KH #"=w712) -> (w711:T23)
        n358 = Unbundle By Name(w711) -> ("KH"=w710:T4)
        n359 = local write "KH"(w710) -> ()
        n360 = call <vilib>:"Add State(s) to Queue__jki_lib_state_machine.vi"("State(s) in (\"\")"=w727) -> ("States Out"=w726:string)  [unwired: 14 in]
      }
      frame "Metadata: Update AI" {
        n361 = local read "Lockin"() -> (w773:T6)
        n362 = Unbundle By Name(w773) -> ("Electrode"=w778:string[], "Label"=w783:u16[], "Electrode Config"=w782:T5[], "AI"=w775:u32[])
        n363 = Empty Array?(array=w775) -> (empty?=w776:bool)
        n364 = case shown="False" w776 {
          tunnel: [w797 string[] [] ("Electrode")] -> w784
          tunnel: w783 -> [w789 _]
          tunnel: w782 -> [w796 _]
          tunnel: [w795 w826] -> w781
          tunnel: w775 -> [w791 _]
          tunnel: [w790 w829] -> w780
          tunnel: [w794 u16[] [] ("Label")] -> w779
          tunnel: w778 -> [w792 _]
          tunnel: w777 -> [w793 w829]
          tunnel: [w791 u32[] [] ("AI")] -> w774
          frame False {
            n365 = Empty Array?(array=w789) -> (empty?=w788:bool)
            n366 = case shown="False" w788 {
              tunnel: [w812 w821] -> w797
              tunnel: w789 -> [w808 w822]
              tunnel: w796 -> [w807 w823]
              tunnel: [w806 w816] -> w795
              tunnel: [w805 w818] -> w794
              tunnel: w793 -> [w804 w813]
              tunnel: w792 -> [w800 w824]
              tunnel: w791 -> [w799 w815]
              tunnel: [w798 w813] -> w790
              frame False {
                n367 = call "Initialize KH Array.vi"("KH #"=w799, "Control in"=w800) -> ("Control out"=w811:variant)  [unwired: 9 in]
                n368 = call "Initialize KH Array.vi"("KH #"=w799, "Control in"=w808) -> ("Control out"=w810:variant)  [unwired: 9 in]
                n369 = call "Initialize KH Array.vi"("KH #"=w799, "Control in"=w807) -> ("Control out"=w809:variant)  [unwired: 9 in]
                n370 = Variant To Data(error in=w804, type=w800, Variant=w811) -> (data=w812:string[], error out=w803:errorcluster)
                n371 = Variant To Data(error in=w804, type=w808, Variant=w810) -> (data=w805:u16[], error out=w802:errorcluster)
                n372 = Variant To Data(error in=w804, type=w807, Variant=w809) -> (data=w806:T5[], error out=w801:errorcluster)
                n373 = Merge Errors(w803, w802, w801) -> (w798:errorcluster)
              }
              frame True {
                n374 = Array Size(array=w815) -> (size(s)=w814:i32)
                n375 = Index Array(array=w822) -> (element=w819:u16)  [unwired: 1 in]
                n376 = Index Array(array=w823) -> (element=w817:T5)  [unwired: 1 in]
                n377 = Index Array(array=w824) -> (element=w820:string)  [unwired: 1 in]
                n378 = Initialize Array(w820, w814) -> (w821:string[])
                n379 = Initialize Array(w819, w814) -> (w818:u16[])
                n380 = Initialize Array(w817, w814) -> (w816:T5[])
              }
            }
          }
          frame True {
            w826 = T1[] [] items=["OFF", "SE+", "SE-", "DIFF"] ("Electrode Config")
          }
        }
        n381 = Bundle By Name(cluster=w785, "Lockin.Electrode"=w784, "Lockin.Label"=w779, "Lockin.Electrode Config"=w781, "Lockin.AI"=w774) -> (w771:T23)
        n382 = Unbundle By Name(w771) -> ("Lockin"=w772:T6)
        n383 = local write "Lockin"(w772) -> ()
        n384 = call <vilib>:"Add State(s) to Queue__jki_lib_state_machine.vi"("State(s) in (\"\")"=w787) -> ("States Out"=w786:string)  [unwired: 14 in]
      }
      frame "Metadata: Build Path" {
        n385 = Unbundle By Name(w838) -> ("Experiment.Device"=w836:string)
        n386 = Build Path(base path="Path", name or relative path=w836) -> (appended path=w835:path)
        n387 = call <vilib>:"Create Directory Recursive.vi"("error in (no error)"=w834, "directory"=w835) -> ("error out"=w833:errorcluster, "directory copy"=w832:path)  [unwired: 3 in, 1 out]
        "Device Folder" <- w832
        n388 = Bundle By Name(cluster=w838, "Experiment.Device Path"=w832) -> (w837:T23)
        n389 = call <vilib>:"Add State(s) to Queue__jki_lib_state_machine.vi"("State(s) in (\"\")"=w840) -> ("States Out"=w839:string)  [unwired: 14 in]
      }
      frame "Metadata: Update Control Experiment Wire" {
        # "IS Control Experiment Class wire"
        # "Not on Control Experiment Class wire"
        n390 = Unbundle By Name(w846) -> ("C.E."=w844:refnum<class "Control Experiment.lvclass">, "Experiment"=w848:T17, "Wiring Configuration"=w847:T20)
        n391 = Bundle By Name(cluster=w844, "Experiment"=w848, "Wiring Configuration"=w847) -> (w842:refnum<class "Control Experiment.lvclass">)
        n392 = Bundle By Name(cluster=w846, "C.E."=w842) -> (w845:T23)
        n393 = call <vilib>:"Add State(s) to Queue__jki_lib_state_machine.vi"("State(s) in (\"\")"=w850) -> ("States Out"=w849:string)  [unwired: 14 in]
      }
      frame "Metadata: Update Comments" {
        n394 = Unbundle By Name(w860) -> ("C.E."=w856:refnum<class "Control Experiment.lvclass">)
        n395 = call "Generate Comments.vi"("error in (no error)"=w854, "Control Experiment"=w856) -> ("error out"=w852:errorcluster, "Control Experiment out"=w855:refnum<class "Control Experiment.lvclass">)  [unwired: 6 in, 1 out]
        n396 = call "Read Comments.vi"("error in (no error)"=w852, "Control Experiment in"=w855) -> ("error out"=w853:errorcluster, "Comments"=→"Comments":string, "Control Experiment out"=w857:refnum<class "Control Experiment.lvclass">)  [unwired: 7 in]
        n397 = Bundle By Name(cluster=w860, "C.E."=w857) -> (w859:T23)
        n398 = call <vilib>:"Add State(s) to Queue__jki_lib_state_machine.vi"("State(s) in (\"\")"=w862) -> ("States Out"=w861:string)  [unwired: 14 in]
      }
      frame "Metadata: Write JSON" {
        w874 = T32 {"Device"={"Device"="", "User"="", "Time"="", "Computer Name"=""}, "Wiring"={"Lockin Ch"=[], "KH Electrodes"=[], "KH Labels"=[], "Other Electrodes"=[], "Other Labels"=[]}}  # Control Experiment JSON
        n399 = Unbundle By Name(w870) -> ("C.E."=w868:refnum<class "Control Experiment.lvclass">, "Experiment.Device"=w882:string, "Experiment.User"=w873:string)
        n400 = Unbundle By Name(w870) -> ("Lockin.AI"=w881:u32[], "Wiring Configuration.KH.Electrodes"=w880:string[], "Wiring Configuration.KH.Labels"=w879:string[], "Wiring Configuration.not KH.Electrodes"=w877:string[], "Wiring Configuration.not KH.Labels"=w876:string[])
        n401 = call "Get Date Time ISO.vi"() -> ("ISO 8601 date-time string"=w875:string)  [unwired: 9 in, 2 out]
        n402 = call "Get Computer Name.vi"() -> ("name"=w878:string)  [unwired: 10 in, 1 out]
        n403 = Bundle By Name(cluster=w874, "Device.Device"=w882, "Device.User"=w873, "Device.Time"=w875, "Device.Computer Name"=w878) -> (w864:T32)
        n404 = Bundle By Name(cluster=w864, "Wiring.Lockin Ch"=w881, "Wiring.KH Electrodes"=w880, "Wiring.KH Labels"=w879, "Wiring.Other Electrodes"=w877, "Wiring.Other Labels"=w876) -> (w869:T32)
        n405 = call "To JSON Text.vim"("error in (no error)"=w872, "Anything"=w869) -> ("error out"=w866:errorcluster, "<JSON>"=w865:string)  [unwired: 8 in]
        "JSON String" <- w865
        n406 = Bundle By Name(cluster=w868, "json"=w865) -> (w867:refnum<class "Control Experiment.lvclass">)
        n407 = Bundle By Name(cluster=w870, "C.E."=w867) -> (w871:T23)
        n408 = call <vilib>:"Add State(s) to Queue__jki_lib_state_machine.vi"("State(s) in (\"\")"=w884) -> ("States Out"=w883:string)  [unwired: 14 in]
      }
      frame "Metadata: Write FGV" {
        n409 = Unbundle By Name(w890) -> ("C.E."=w888:refnum<class "Control Experiment.lvclass">)
        n410 = call "Control Experiment FGV.vi"("Function"=enum16{"read", "write"}."write", "error in (no error)"=w886, "Control Experiment.lvclass"=w888) -> ("error out"=w887:errorcluster)  [unwired: 7 in, 1 out]
        n411 = call <vilib>:"Add State(s) to Queue__jki_lib_state_machine.vi"("State(s) in (\"\")"=w892) -> ("States Out"=w891:string)  [unwired: 14 in]
      }
      frame "Metadata: Read FGV" {
        n412 = call "Control Experiment FGV.vi"("Function"=enum16{"read", "write"}."read", "error in (no error)"=w897) -> ("error out"=w898:errorcluster, "Control Experiment.lvclass out"=w896:refnum<class "Control Experiment.lvclass">)  [unwired: 8 in]
        n413 = Bundle By Name(cluster=w894, "C.E."=w896) -> (w895:T23)
        n414 = call <vilib>:"Add State(s) to Queue__jki_lib_state_machine.vi"("State(s) in (\"\")"=w901) -> ("States Out"=w900:string)  [unwired: 14 in]
      }
      frame "---------- KH ----------" {
        # "Do not put any code in this frame.\n(it is a separator no-op)"
        n415 = call <vilib>:"Add State(s) to Queue__jki_lib_state_machine.vi"("State(s) in (\"\")"=w906) -> ("States Out"=w905:string)  [unwired: 14 in]
      }
      frame "KH: set KH 0" {
        # "#KHChassis"
        # "initialize the Channel Settings array"
        n416 = Initialize Array(T13 {"channel"=0, "gain"=enum."10", "input"=enum."SE+", "shunt"=enum."50", "couple"=enum."DC", "filter"=enum."OFF"} ("Channel Settings"), 8 ("dimension size")) -> (w914:T13[])
        n417 = Bundle(w914) -> (w913:cluster{T13[]})  [unwired: 1 in]
        n418 = for {
          N: "KH Chassis" -> [_]
          tunnel: [w925] -> w910 mode=concatenating
          shift-right: [w923] -> w912
          shift-left: w909 -> [w924]
          i -> [w927]
          n419 = call "Number to Letter.vi"("Number"=w927) -> ("Letter"=w926:string)
          n420 = for {
            N: 8 -> [_]
            tunnel: w926 -> [w932]
            tunnel: [w931] -> w925 mode=indexing
            shift-right: [w929] -> w923
            shift-left: w924 -> [w930]
            i -> [w934]
            n421 = Increment(x=w934) -> (x+1=w928:i32)
            n422 = Format Into String(format string="%s %d", error in=w930, w932, w928) -> (resulting string=w931:string, error out=w929:errorcluster)  [unwired: 1 in]
          }
        }
        n423 = Initialize Array(w913, "KH Chassis") -> (w917:cluster{T13[]}[])
        n424 = Bundle By Name(cluster=w919, "Channel Settings"=w917) -> (w918:T23)
        n425 = property on="Ring" class="Ring (strict)"(error in=w912, "Strings []"=w910) -> (error out=w911:errorcluster)  [unwired: 1 in, 1 out]
        n426 = call <vilib>:"Add State(s) to Queue__jki_lib_state_machine.vi"("State(s) in (\"\")"=w921) -> ("States Out"=w920:string)  [unwired: 14 in]
      }
      frame "KH: set KH 1" {
        n427 = Unbundle By Name(w947) -> ("Channel Settings"=w936:cluster{"Channel Setting":T21}[], "KH.KH #"=w949:u16[], "KH.KH Gain"=w952:T2[], "Lockin.Electrode Config"=w950:T5[], "KH.KH Shunt Resistor"=w951:T3[], "KH Configuration"=w948:T7)
        n428 = local read "DC Coupled"() -> (w938:bool)
        n429 = local read "BW Filter"() -> (w937:bool)
        n430 = for {
          tunnel: w950 -> [w977] mode=indexing
          tunnel: w952 -> [w976] mode=indexing
          tunnel: w951 -> [w975] mode=indexing
          tunnel: w949 -> [w971] mode=indexing
          tunnel: [w980] -> w943 mode=indexing
          tunnel: w948 -> [w979]
          tunnel: [w978] -> w941 mode=indexing
          tunnel: [w974] -> w942 mode=indexing
          shift-right: [w967] -> w945
          shift-left: w936 -> [w968]
          tunnel: w938 -> [w963]
          tunnel: w937 -> [w958]
          n431 = property on="Ring" class="Ring (strict)"() -> ("Strings []"=w973:string[])  [unwired: 2 in, 2 out]
          n432 = case shown="\"No Selection\", Default" w979 {
            tunnel: w977 -> [w999 _ _]
            tunnel: [w1004 Input--Enum."OFF" ("Input Config") Input--Enum."DIFF" ("Input Config")] -> w974
            tunnel: w976 -> [w1003 w1022 w1025]
            tunnel: [w1002 w1022 w1025] -> w978
            tunnel: w975 -> [w1001 _ w1023]
            tunnel: [w1000 shunt--enum."Open" ("Shunt Resistor") w1023] -> w980
            frame "No Selection", Default {
              n433 = case shown="\"Ground\", Default" w999 {
                tunnel: [Input--Enum."OFF" ("Input Config") Input--Enum."DIFF" ("Input Config") Input--Enum."SE+" ("Input Config") Input--Enum."DIFF" ("Input Config") Input--Enum."DIFF" ("Input Config")] -> w1004
                tunnel: [shunt--enum."Open" ("Shunt Resistor") w1008 shunt--enum."Open" ("Shunt Resistor") shunt--enum."Open" ("Shunt Resistor") w1017] -> w1000
                tunnel: w1003 -> [w1005 w1009 w1012 w1016 w1018]
                tunnel: [w1005 w1009 w1012 w1016 w1018] -> w1002
                tunnel: w1001 -> [_ w1008 _ _ w1017]
                frame "Ground", Default {
                }
                frame "Current" {
                }
                frame "Voltage (SE)" {
                }
                frame "Voltage (Diff)" {
                }
                frame "Gate" {
                }
              }
            }
            frame "All Ground" {
            }
            frame "All Differential" {
            }
          }
          n434 = To Long Integer(number=w971) -> (32bit integer=w972:i32)
          n435 = Index Array(array=w973, index=w972) -> (element=w970:string)
          n436 = Select(t=couple--Enum."DC" ("Coupling"), s=w963, f=couple--Enum."AC" ("Coupling")) -> (s? t:f=w960:T15)
          n437 = Scan From String(format string="%s %d", input string=w970) -> (error out=w964:errorcluster, output 1=w966:string, output 2=w965:i32)  [unwired: 4 in, 2 out]
          n438 = Select(t=Filter--Enum."ON" ("Bandwidth Filter"), s=w958, f=Filter--Enum."OFF" ("Bandwidth Filter")) -> (s? t:f=w956:T16)
          n439 = case shown="No Error" w964 {
            tunnel: w980 -> [w997 _]
            tunnel: w978 -> [w996 _]
            tunnel: w974 -> [w995 _]
            tunnel: w968 -> [w987 w998]
            tunnel: [w986 w998] -> w967
            tunnel: w966 -> [w985 _]
            tunnel: w965 -> [w981 _]
            tunnel: w960 -> [w984 _]
            tunnel: w956 -> [w983 _]
            frame No Error {
              n440 = call "Letter to Number.vi"("Letter"=w985) -> ("Number"=w988:i32)
              n441 = Decrement(x=w981) -> (x-1=w982:i32)
              n442 = Index Array(array=w987, index=w988) -> (element=w993:cluster{"Channel Setting":T21})
              n443 = Unbundle(w993) -> ("Channel Setting"=w992:T21)
              n444 = Index Array(array=w992, index=w982) -> (element=w991:T13)
              n445 = Bundle By Name(cluster=w991, "channel"=w981, "gain"=w996, "input"=w995, "shunt"=w997, "couple"=w984, "filter"=w983) -> (w990:T13)
              n446 = Replace Array Subset(array=w992, new element=w990, index=w982) -> (w994:T21)
              n447 = Bundle("Channel Setting"=w994) -> (w989:cluster{"Channel Setting":T21})  [unwired: 1 in]
              n448 = Replace Array Subset(array=w987, new element=w989, index=w988) -> (w986:cluster{"Channel Setting":T21}[])
            }
            frame Error {
            }
          }
        }
        n449 = local write "KH Configuration"(T7."No Selection" ("KH All Buttons")) -> ()
        n450 = Bundle By Name(cluster=w947, "Channel Settings"=w945, "KH.KH Gain"=w941, "KH.KH Configuration"=w942, "KH.KH Shunt Resistor"=w943) -> (w953:T23)
        n451 = local read "KH"() -> (w944:T4)
        n452 = Bundle By Name(cluster=w944, "KH Gain"=w941, "KH Configuration"=w942, "KH Shunt Resistor"=w943) -> (w940:T4)
        n453 = local write "KH"(w940) -> ()
        n454 = call <vilib>:"Add State(s) to Queue__jki_lib_state_machine.vi"("State(s) in (\"\")"=w955) -> ("States Out"=w954:string)  [unwired: 14 in]
      }
      frame "KH: set KH 2" {
        # "getAllChannels"
        # "setAllChannels"
        n455 = Unbundle By Name(w1042) -> ("C.E."=w1030:refnum<class "Control Experiment.lvclass">)
        n456 = Unbundle By Name(w1042) -> ("Channel Settings"=w1032:cluster{"Channel Setting":T21}[])
        n457 = Unbundle By Name(w1030) -> ("Amplifier"=w1038:refnum<class "Instrument.Amplifier.lvclass">)
        n458 = To More Specific Class(target class=refnum<class "Inst.Krohn-Hite-7008.lvclass"> refnum ("Inst.KH7008.lvlib:Inst.Krohn-Hite-7008.lvclass"), reference=w1038) -> (specific class reference=w1036:refnum<class "Inst.Krohn-Hite-7008.lvclass">)  [unwired: 1 in, 1 out]
        n459 = for {
          tunnel: [w1058] -> w1040 mode=indexing
          tunnel: w1032 -> [w1061] mode=indexing
          tunnel: w1036 -> [w1053]
          tunnel: [w1056] -> w1034
          shift-right: [w1054] -> w1033
          shift-left: w1037 -> [w1050]
          i -> [w1049]
          n460 = Increment(x=w1049) -> (x+1=w1048:i32)
          n461 = Unbundle(w1061) -> ("Channel Setting"=w1059:T21)
          n462 = call-dynamic "Inst.KH7008.Open.vi"("error in (no error)"=w1050, "index"=w1048, "Inst.Krohn-Hite-7008 in"=w1053) -> ("error out"=w1051:errorcluster, "Inst.Krohn-Hite-7008 out"=w1052:refnum<class "Inst.Krohn-Hite-7008.lvclass">)  [unwired: 7 in]
          n463 = call-dynamic "Inst.KH7008.setAllChannels.vi"("error in (no error)"=w1051, "allChannelProperties"=w1059, "Inst.Krohn-Hite-7008 in"=w1052) -> ("error out"=w1063:errorcluster, "Inst.Krohn-Hite-7008 out"=w1062:refnum<class "Inst.Krohn-Hite-7008.lvclass">)  [unwired: 7 in]
          n464 = for {
            N: 10 -> [_]
            tunnel: w1062 -> [w1075]
            tunnel: [w1076] -> w1057
            tunnel: w1059 -> [w1070]
            tunnel: [w1064] -> w1058
            shift-right: [w1074] -> w1055
            shift-left: w1063 -> [w1068]
            i -> [w1065]
            stop <- w1069 stop-if-true
            n465 = Equal To 0?(x=w1065) -> (x = 0?=w1072:bool)
            n466 = Select(t=w1065, s=w1072, f=100) -> (s? t:f=w1066:i32)
            n467 = call <userlib>:"Wait (ms)__ogtk.vi"("error in (no error)"=w1068, "milliseconds to wait"=w1066) -> ("error out"=w1073:errorcluster)  [unwired: 8 in, 1 out]
            n468 = call-dynamic "Inst.KH7008.getAllChannels.vi"("error in (no error)"=w1073, "Inst.Krohn-Hite-7008 in"=w1075) -> ("error out"=w1074:errorcluster, "allChannelProperties"=w1067:T21, "Inst.Krohn-Hite-7008 out"=w1076:refnum<class "Inst.Krohn-Hite-7008.lvclass">)  [unwired: 7 in]
            n469 = Equal?(x=w1067, y=w1070) -> (x = y?=w1069:bool)
            n470 = Bundle("allChannelProperties"=w1067) -> (w1064:cluster{"allChannelProperties":T21})  [unwired: 1 in]
          }
          n471 = call-dynamic "Close.vi"("error in (no error)"=w1055, "Inst.Krohn-Hite-7008 in"=w1057) -> ("error out"=w1054:errorcluster, "Inst.Krohn-Hite-7008 out"=w1056:refnum<class "Inst.Krohn-Hite-7008.lvclass">)  [unwired: 8 in]
        }
        n472 = Bundle By Name(cluster=w1030, "Amplifier"=w1034) -> (w1028:refnum<class "Control Experiment.lvclass">)
        n473 = local read "Gain"() -> (w1043:dbl[])
        n474 = call "Multiply Gains.vi"("Other Gain"=w1043, "Array"=w1040) -> ("Gain x Other Gain"=w1031:dbl[])
        n475 = Unbundle By Name(w1028) -> ("DAQ"=w1035:refnum<class "Instrument.LockinAPI.lvclass">)
        n476 = call-dynamic "setInputGain.vi"("error in (no error)"=w1033, "InputGain"=w1031, "Instrument.LockinAPI in"=w1035) -> ("error out"=w1041:errorcluster, "Instrument.LockinAPI out"=w1029:refnum<class "Instrument.LockinAPI.lvclass">)  [unwired: 7 in]
        n477 = Bundle By Name(cluster=w1028, "DAQ"=w1029) -> (w1027:refnum<class "Control Experiment.lvclass">)
        n478 = Bundle By Name(cluster=w1042, "C.E."=w1027) -> (w1045:T23)
        n479 = call <vilib>:"Clear Errors.vi"("error in (no error)"=w1041) -> ("error out"=w1044:errorcluster)  [unwired: 5 in, 1 out]
        n480 = call <vilib>:"Add State(s) to Queue__jki_lib_state_machine.vi"("State(s) in (\"\")"=w1047) -> ("States Out"=w1046:string)  [unwired: 14 in]
      }
      frame "KH: get KH Number" {
        # "KH: Get KH Number\n(Check how many KH amplifiers are configured"
        n481 = Unbundle By Name(w1087) -> ("C.E."=w1086:refnum<class "Control Experiment.lvclass">)
        n482 = Unbundle By Name(w1086) -> ("Amplifier"=w1089:refnum<class "Instrument.Amplifier.lvclass">)
        n483 = To More Specific Class(target class=refnum<class "Inst.Krohn-Hite-7008.lvclass"> refnum ("Inst.KH7008.lvlib:Inst.Krohn-Hite-7008.lvclass"), reference=w1089) -> (specific class reference=w1088:refnum<class "Inst.Krohn-Hite-7008.lvclass">)  [unwired: 1 in, 1 out]
        n484 = call-dynamic "Inst.KH7008.Open.vi"("error in (no error)"=w1084, "index"=1, "Inst.Krohn-Hite-7008 in"=w1088) -> ("error out"=w1081:errorcluster, "Inst.Krohn-Hite-7008 out"=w1083:refnum<class "Inst.Krohn-Hite-7008.lvclass">)  [unwired: 7 in]
        n485 = case shown="No Error" w1081 {
          selector: w1081 -> [w1095 _]
          tunnel: w1083 -> [w1097 w1098]
          tunnel: [w1096 w1098] -> w1082
          tunnel: [w1094 _] -> w1080
          tunnel: [w1093 0 ("Number of Chassis")] -> w1078
          frame No Error {
            n486 = call-dynamic "Inst.KH7008.getChassis.vi"("error in (no error)"=w1095, "Inst.Krohn-Hite-7008 in"=w1097) -> ("error out"=w1094:errorcluster, "Number of Chassis"=w1093:i32, "Inst.Krohn-Hite-7008 out"=w1096:refnum<class "Inst.Krohn-Hite-7008.lvclass">)  [unwired: 7 in]
          }
          frame Error {
          }
        }
        n487 = local write "KH Chassis"(w1078) -> ()
        n488 = call-dynamic "Close.vi"("error in (no error)"=w1080, "Inst.Krohn-Hite-7008 in"=w1082) -> ("error out"=w1085:errorcluster)  [unwired: 8 in, 1 out]
        n489 = call <vilib>:"Add State(s) to Queue__jki_lib_state_machine.vi"("State(s) in (\"\")"=w1092) -> ("States Out"=w1091:string)  [unwired: 14 in]
      }
      frame "KH: get KH" {
        # "getAllChannels"
        # "setAllChannels"
        n490 = Unbundle By Name(w1109) -> ("C.E."=w1104:refnum<class "Control Experiment.lvclass">)
        n491 = Unbundle By Name(w1104) -> ("Amplifier"=w1107:refnum<class "Instrument.Amplifier.lvclass">)
        n492 = local read "KH Chassis"() -> (w1103:i32)
        n493 = To More Specific Class(target class=refnum<class "Inst.Krohn-Hite-7008.lvclass"> refnum ("Inst.KH7008.lvlib:Inst.Krohn-Hite-7008.lvclass"), reference=w1107) -> (specific class reference=w1105:refnum<class "Inst.Krohn-Hite-7008.lvclass">)  [unwired: 1 in, 1 out]
        n494 = for {
          N: w1103 -> [_]
          tunnel: [w1123] -> w1101 mode=indexing
          tunnel: w1105 -> [w1119]
          tunnel: w1106 -> [w1117]
          tunnel: [w1120] -> w1102
          i -> [w1116]
          n495 = Increment(x=w1116) -> (x+1=w1114:i32)
          n496 = call-dynamic "Inst.KH7008.Open.vi"("error in (no error)"=w1117, "index"=w1114, "Inst.Krohn-Hite-7008 in"=w1119) -> ("error out"=w1118:errorcluster, "Inst.Krohn-Hite-7008 out"=w1124:refnum<class "Inst.Krohn-Hite-7008.lvclass">)  [unwired: 7 in]
          n497 = call-dynamic "Inst.KH7008.getAllChannels.vi"("error in (no error)"=w1118, "Inst.Krohn-Hite-7008 in"=w1124) -> ("error out"=w1121:errorcluster, "allChannelProperties"=w1115:T21, "Inst.Krohn-Hite-7008 out"=w1122:refnum<class "Inst.Krohn-Hite-7008.lvclass">)  [unwired: 7 in]
          n498 = Bundle("allChannelProperties"=w1115) -> (w1123:cluster{"allChannelProperties":T21})  [unwired: 1 in]
          n499 = call-dynamic "Close.vi"("error in (no error)"=w1121, "Inst.Krohn-Hite-7008 in"=w1122) -> ("error out"=w1120:errorcluster)  [unwired: 8 in, 1 out]
        }
        n500 = Bundle By Name(cluster=w1109, "Channel Settings"=w1101) -> (w1111:T23)
        n501 = call <vilib>:"Clear Errors.vi"("error in (no error)"=w1102) -> ("error out"=w1110:errorcluster)  [unwired: 5 in, 1 out]
        n502 = call <vilib>:"Add State(s) to Queue__jki_lib_state_machine.vi"("State(s) in (\"\")"=w1113) -> ("States Out"=w1112:string)  [unwired: 14 in]
      }
      frame "---------- Instruments ----------" {
        # "Do not put any code in this frame.\n(it is a separator no-op)"
        n503 = call <vilib>:"Add State(s) to Queue__jki_lib_state_machine.vi"("State(s) in (\"\")"=w1129) -> ("States Out"=w1128:string)  [unwired: 14 in]
      }
      frame "Instruments: Load Classes" {
        n504 = Unbundle By Name(w1136) -> ("C.E."=w1134:refnum<class "Control Experiment.lvclass">)
        n505 = call "Load Instrument Classes.vi"("error in (no error)"=w1133, "C.E."=w1134) -> ("error out"=w1131:errorcluster, "Control Experiment"=w1132:refnum<class "Control Experiment.lvclass">)  [unwired: 8 in]
        n506 = Bundle By Name(cluster=w1136, "C.E."=w1132) -> (w1135:T23)
        n507 = call <vilib>:"Add State(s) to Queue__jki_lib_state_machine.vi"("State(s) in (\"\")"=w1138) -> ("States Out"=w1137:string)  [unwired: 14 in]
      }
      frame "---------- Instrument ----------" {
        n508 = call <vilib>:"Add State(s) to Queue__jki_lib_state_machine.vi"("State(s) in (\"\")"=w1143) -> ("States Out"=w1142:string)  [unwired: 14 in]
      }
      frame "Instrument: Lockin Status" {
        n509 = Unbundle By Name(w1153) -> ("C.E."=w1151:refnum<class "Control Experiment.lvclass">)
        n510 = Unbundle By Name(w1151) -> ("DAQ"=w1157:refnum<class "Instrument.LockinAPI.lvclass">)
        n511 = call-dynamic "Open.vi"("Instrument in"=w1157) -> ("error out"=w1158:errorcluster, "Instrument out"=w1156:refnum<class "Instrument.LockinAPI.lvclass">)  [unwired: 9 in]
        n512 = call <userlib>:"ACK.vi"("error in (no error)"=w1158, "Instrument in"=w1156) -> ("error out"=w1146:errorcluster, "ACK"=w1155:string, "Instrument out"=w1147:refnum<class "Instrument.LockinAPI.lvclass">)  [unwired: 7 in]
        n513 = case shown="Default" w1155 {
          tunnel: [w1171 w1176] -> w1152
          tunnel: w1151 -> [w1171 w1176]
          tunnel: [TRUE ("Lockin?") FALSE ("Lockin?")] -> w1150
          tunnel: [FALSE ("Lockin?") TRUE ("Lockin?")] -> w1149
          tunnel: w1147 -> [w1168 w1173]
          tunnel: w1146 -> [w1167 w1172]
          tunnel: [w1166 w1172] -> w1145
          tunnel: [w1165 w1173] -> w1144
          frame Default {
            n514 = call <userlib>:"IDN.vi"("error in (no error)"=w1167, "Instrument in"=w1168) -> ("error out"=w1166:errorcluster, "IDN"=w1164:T33, "Instrument in"=w1165:refnum<class "Instrument.LockinAPI.lvclass">)  [unwired: 7 in]
            n515 = Unbundle By Name(w1164) -> ("serial"=→"MCL S/N":string)
          }
          frame "" {
          }
        }
        n516 = call-dynamic "Close.vi"("error in (no error)"=w1145, "Instrument in"=w1144) -> ()  [unwired: 8 in, 2 out]
        n517 = property on="Lockin?" class="Bool (strict)"("Value"=w1150, "Blinking"=w1149) -> ()  [unwired: 2 in, 2 out]
        n518 = Bundle By Name(cluster=w1153, "C.E."=w1152) -> (w1154:T23)
        n519 = call <vilib>:"Add State(s) to Queue__jki_lib_state_machine.vi"("State(s) in Front (\"\")"="" ("State(s) in Front (\"\")"), "State(s) in (\"\")"=w1162) -> ("States Out"=w1161:string)  [unwired: 13 in]
      }
      frame "Instrument: KH Status" {
        n520 = Unbundle By Name(w1193) -> ("C.E."=w1188:refnum<class "Control Experiment.lvclass">)
        n521 = Unbundle By Name(w1188) -> ("Amplifier"=w1189:refnum<class "Instrument.Amplifier.lvclass">)
        n522 = To More Specific Class(target class=refnum<class "Inst.Krohn-Hite-7008.lvclass"> refnum ("Inst.KH7008.lvlib:Inst.Krohn-Hite-7008.lvclass"), reference=w1189) -> (specific class reference=w1187:refnum<class "Inst.Krohn-Hite-7008.lvclass">)  [unwired: 1 in, 1 out]
        n523 = call-dynamic "Inst.KH7008.Open.vi"("index"=1, "Inst.Krohn-Hite-7008 in"=w1187) -> ("error out"=w1178:errorcluster, "Inst.Krohn-Hite-7008 out"=w1179:refnum<class "Inst.Krohn-Hite-7008.lvclass">)  [unwired: 8 in]
        n524 = call <userlib>:"ACK.vi"("error in (no error)"=w1178, "Instrument in"=w1179) -> ("error out"=w1182:errorcluster, "ACK"=w1186:string, "Instrument out"=w1183:refnum<class "Inst.Krohn-Hite-7008.lvclass">)  [unwired: 7 in]
        n525 = case shown="Default" w1186 {
          tunnel: [w1204 w1210] -> w1192
          tunnel: w1188 -> [w1204 w1210]
          tunnel: ["" ("State(s) in Front (\"\")") "KH: get KH Number\nInstrument: get KH SN\nUI: SR Disable" ("State(s) in Front (\"\")")] -> w1191
          tunnel: [FALSE ("KH?") TRUE ("KH?")] -> w1185
          tunnel: [TRUE ("KH?") FALSE ("KH?")] -> w1184
          tunnel: w1183 -> [w1202 w1205]
          tunnel: w1182 -> [w1201 w1206]
          tunnel: [w1201 w1206] -> w1181
          tunnel: [w1202 w1205] -> w1180
          frame "" {
          }
          frame Default {
          }
        }
        n526 = property on="KH?" class="Bool (strict)"("Value"=w1185, "Blinking"=w1184) -> ()  [unwired: 2 in, 2 out]
        n527 = call-dynamic "Close.vi"("error in (no error)"=w1181, "Inst.Krohn-Hite-7008 in"=w1180) -> ()  [unwired: 8 in, 2 out]
        n528 = Bundle By Name(cluster=w1193, "C.E."=w1192) -> (w1194:T23)
        n529 = call <vilib>:"Add State(s) to Queue__jki_lib_state_machine.vi"("State(s) in Front (\"\")"=w1191, "State(s) in (\"\")"=w1198) -> ("States Out"=w1197:string)  [unwired: 13 in]
      }
      frame "Instrument: get KH SN" {
        n530 = Unbundle By Name(w1221) -> ("C.E."=w1216:refnum<class "Control Experiment.lvclass">)
        n531 = Unbundle By Name(w1216) -> ("Amplifier"=w1217:refnum<class "Instrument.Amplifier.lvclass">)
        n532 = local read "KH Chassis"() -> (w1214:i32)
        n533 = To More Specific Class(target class=refnum<class "Inst.Krohn-Hite-7008.lvclass"> refnum ("Inst.KH7008.lvlib:Inst.Krohn-Hite-7008.lvclass"), reference=w1217) -> (specific class reference=w1215:refnum<class "Inst.Krohn-Hite-7008.lvclass">)  [unwired: 1 in, 1 out]
        n534 = for {
          N: w1214 -> [_]
          tunnel: [w1238] -> w1219
          tunnel: w1215 -> [w1232]
          shift-right: [w1239] -> w1220
          shift-left: w1216 -> [w1237]
          tunnel: [w1227] -> w1213 mode=indexing
          i -> [w1229]
          n535 = Increment(x=w1229) -> (x+1=w1228:i32)
          n536 = call-dynamic "Inst.KH7008.Open.vi"("index"=w1228, "Inst.Krohn-Hite-7008 in"=w1232) -> ("error out"=w1230:errorcluster, "Inst.Krohn-Hite-7008 out"=w1231:refnum<class "Inst.Krohn-Hite-7008.lvclass">)  [unwired: 8 in]
          n537 = call <userlib>:"ACK.vi"("error in (no error)"=w1230, "Instrument in"=w1231) -> ("error out"=w1235:errorcluster, "ACK"=w1240:string, "Instrument out"=w1236:refnum<class "Inst.Krohn-Hite-7008.lvclass">)  [unwired: 7 in]
          n538 = case shown="\"\"" w1240 {
            tunnel: [w1244 w1252] -> w1239
            tunnel: w1237 -> [w1244 w1252]
            tunnel: [w1241 "" ("State(s) in Front (\"\")")] -> w1238
            tunnel: w1236 -> [w1243 w1250]
            tunnel: w1235 -> [w1242 w1249]
            tunnel: [w1242 w1248] -> w1234
            tunnel: [w1243 w1247] -> w1233
            tunnel: [w1241 w1245] -> w1227
            frame "" {
              w1241 = "" ("State(s) in Front (\"\")")
            }
            frame Default {
              n539 = call <userlib>:"IDN.vi"("error in (no error)"=w1249, "Instrument in"=w1250) -> ("error out"=w1248:errorcluster, "IDN"=w1246:T33, "Instrument in"=w1247:refnum<class "Inst.Krohn-Hite-7008.lvclass">)  [unwired: 7 in]
              n540 = Unbundle By Name(w1246) -> ("serial"=w1245:string)
            }
          }
          n541 = call-dynamic "Close.vi"("error in (no error)"=w1234, "Inst.Krohn-Hite-7008 in"=w1233) -> ()  [unwired: 8 in, 2 out]
        }
        n542 = call <vilib>:"1D String Array to Delimited String.vi"("delimiter"=",", "string array"=w1213) -> ("delimited string"=→"KH S/N":string)  [unwired: 9 in]
        n543 = Bundle By Name(cluster=w1221, "C.E."=w1220) -> (w1222:T23)
        n544 = call <vilib>:"Add State(s) to Queue__jki_lib_state_machine.vi"("State(s) in Front (\"\")"=w1219, "State(s) in (\"\")"=w1226) -> ("States Out"=w1225:string)  [unwired: 13 in]
      }
      frame "Instrument: Open Lockin" {
        n545 = call "Open Lockin.vi"("error in (no error)"=w1255) -> ("error out"=w1254:errorcluster)  [unwired: 10 in]
        n546 = call <vilib>:"Add State(s) to Queue__jki_lib_state_machine.vi"("State(s) in (\"\")"=w1258) -> ("States Out"=w1257:string)  [unwired: 14 in]
      }
      frame "Instrument: Open KH7008" {
        n547 = call "Open KH7008.vi"("error in (no error)"=w1261) -> ("error out"=w1260:errorcluster)  [unwired: 10 in]
        n548 = call <vilib>:"Add State(s) to Queue__jki_lib_state_machine.vi"("State(s) in (\"\")"=w1264) -> ("States Out"=w1263:string)  [unwired: 14 in]
      }
      frame "---------- Transport Server ----------" {
        # "Do not put any code in this frame.\n(it is a separator no-op)"
        n549 = call <vilib>:"Add State(s) to Queue__jki_lib_state_machine.vi"("State(s) in (\"\")"=w1269) -> ("States Out"=w1268:string)  [unwired: 14 in]
      }
      frame "Transport Server: Create" {
        n550 = Unbundle By Name(w1277) -> ("Transport-Server"=w1275:refnum<class "Inst.Transport.lvclass">)
        n551 = call <userlib>:"Create Instrument SMO.vi"("error in (no error)"=w1273, "Debug Mode? [F]"=FALSE, "Configuration Window? [T]"=FALSE, "Instrument in"=w1275) -> ("error out"=w1271:errorcluster, "Instrument out"=w1274:refnum<class "Inst.Transport.lvclass">)  [unwired: 6 in]
        n552 = Bundle By Name(cluster=w1277, "Transport-Server"=w1274) -> (w1278:T23)
        n553 = call <vilib>:"Add State(s) to Queue__jki_lib_state_machine.vi"("State(s) in (\"\")"=w1280) -> ("States Out"=w1279:string)  [unwired: 14 in]
      }
      frame "Transport Server: Start" {
        n554 = Unbundle By Name(w1282) -> ("Transport-Server"=w1287:refnum<class "Inst.Transport.lvclass">)
        n555 = call <vilib>:"Start.vi"("error in (no error)"=w1284, "SMO"=w1287) -> ("error out"=w1285:errorcluster, "SMO out"=w1286:refnum<class "Inst.Transport.lvclass">)  [unwired: 8 in]
        n556 = Bundle By Name(cluster=w1282, "Transport-Server"=w1286) -> (w1283:T23)
        n557 = call <vilib>:"Add State(s) to Queue__jki_lib_state_machine.vi"("State(s) in (\"\")"=w1289) -> ("States Out"=w1288:string)  [unwired: 14 in]
      }
      frame "Transport Server: Stop" {
        n558 = Unbundle By Name(w1294) -> ("Transport-Server"=w1292:refnum<class "Inst.Transport.lvclass">)
        n559 = call <vilib>:"Stop.vi"("error in (no error)"=w1291, "SMO"=w1292) -> ("error out"=w1290:errorcluster, "SMO out"=w1296:refnum<class "Inst.Transport.lvclass">)  [unwired: 8 in]
        n560 = Bundle By Name(cluster=w1294, "Transport-Server"=w1296) -> (w1295:T23)
        n561 = call <vilib>:"Add State(s) to Queue__jki_lib_state_machine.vi"("State(s) in (\"\")"=w1298) -> ("States Out"=w1297:string)  [unwired: 14 in]
      }
      frame "Transport Server: Destroy" {
        n562 = Unbundle By Name(w1301) -> ("Transport-Server"=w1305:refnum<class "Inst.Transport.lvclass">)
        n563 = call <vilib>:"Destroy.vi"("error in (no error)"=w1303, "SMO"=w1305) -> ("error out"=w1304:errorcluster)  [unwired: 9 in]
        n564 = Bundle By Name(cluster=w1301, "Transport-Server"=refnum<class "Inst.Transport.lvclass"> refnum ("Inst.Transport")) -> (w1302:T23)
        n565 = call <vilib>:"Add State(s) to Queue__jki_lib_state_machine.vi"("State(s) in (\"\")"=w1307) -> ("States Out"=w1306:string)  [unwired: 14 in]
      }
      frame "Transport Server: Show" {
        # "Do not put any code in this frame.\n(it is a separator no-op)"
        n566 = Unbundle By Name(w1312) -> ("Transport-Server"=w1308:refnum<class "Inst.Transport.lvclass">)
        n567 = call "showUI.vi"("error in (no error)"=w1310, "Inst.Transport in"=w1308) -> ("error out"=w1311:errorcluster)  [unwired: 8 in, 1 out]
        n568 = Bundle By Name(cluster=w1312, "Transport-Server"=w1308) -> (w1313:T23)
        n569 = call <vilib>:"Add State(s) to Queue__jki_lib_state_machine.vi"("State(s) in (\"\")"=w1315) -> ("States Out"=w1314:string)  [unwired: 14 in]
      }
      frame "Transport Server: Hide" {
        # "Do not put any code in this frame.\n(it is a separator no-op)"
        n570 = Unbundle By Name(w1320) -> ("Transport-Server"=w1316:refnum<class "Inst.Transport.lvclass">)
        n571 = call "hideUI.vi"("error in (no error)"=w1318, "Inst.Transport in"=w1316) -> ("error out"=w1319:errorcluster)  [unwired: 8 in, 1 out]
        n572 = Bundle By Name(cluster=w1320, "Transport-Server"=w1316) -> (w1321:T23)
        n573 = call <vilib>:"Add State(s) to Queue__jki_lib_state_machine.vi"("State(s) in (\"\")"=w1323) -> ("States Out"=w1322:string)  [unwired: 14 in]
      }
      frame "---------- PGSQL ----------" {
        # "Do not put any code in this frame.\n(it is a separator no-op)"
        n574 = call <vilib>:"Add State(s) to Queue__jki_lib_state_machine.vi"("State(s) in (\"\")"=w1328) -> ("States Out"=w1327:string)  [unwired: 14 in]
      }
      frame "PGSQL: Write" {
        w1339 = "" ("f")
        n575 = Unbundle By Name(w1342) -> ("Experiment.Device"=w1331:string, "Experiment.User"=w1341:string, "Experiment.Instrument"=w1340:string)
        n576 = local read "I'm Finished Taking Data!"() -> (w1332:bool)
        n577 = Not(x=w1332) -> (.not. x?=w1338:bool)
        n578 = Select(t=w1341, s=w1338, f=w1339) -> (s? t:f=w1336:string)
        n579 = Select(t=w1340, s=w1338, f=w1339) -> (s? t:f=w1337:string)
        n580 = local read "MCL S/N"() -> (w1330:string)
        n581 = local read "KH S/N"() -> (w1329:string)
        n582 = call "DB Set Measurement.vi"("KH serial number"=w1329, "lockin serial number"=w1330, "device"=w1331, "error in (no error)"=w1335, "Station"=w1337, "User"=w1336) -> ("error out"=w1334:errorcluster)  [unwired: 5 in]
        n583 = call <vilib>:"Add State(s) to Queue__jki_lib_state_machine.vi"("State(s) in (\"\")"=w1344) -> ("States Out"=w1343:string)  [unwired: 14 in]
      }
      frame "---------- Sequence ----------" {
        # "Do not put any code in this frame.\n(it is a separator no-op)"
        n584 = call <vilib>:"Add State(s) to Queue__jki_lib_state_machine.vi"("State(s) in (\"\")"=w1349) -> ("States Out"=w1348:string)  [unwired: 14 in]
      }
      frame "Sequence: Wait" {
        # "Do not put any code in this frame.\n(it is a separator no-op)"
        n585 = Scan From String(input string=w1352, default 1=u32 0 ("milliseconds to wait")) -> (output 1=w1351:u32)  [unwired: 3 in, 3 out]
        n586 = Wait (ms)(milliseconds to wait=w1351) -> ()  [unwired: 1 out]
        n587 = call <vilib>:"Add State(s) to Queue__jki_lib_state_machine.vi"("State(s) in (\"\")"=w1357) -> ("States Out"=w1356:string)  [unwired: 14 in]
      }
    }
  }
  "Error Out" <- w2
  n588 = Unbundle By Name(w6) -> ("C.E."=→"Control Experiment":refnum<class "Control Experiment.lvclass">)
